vi "Kinect MVMT (state machine).vi"() -> ()   [LabVIEW 2011]
uses:
  Mouse Data Cluster.ctl
  <vilib>/vision/Image Controls.llb/IMAQ Image.ctl
  <vilib>/vision/NI_Vision_Development_Module.lvlib
panel:
  out "concatenated string 2":string
  out "Experiment Metadata":string
  in  "Experiment Metadata":i32(listbox)
  in  "Experiment File":path=path "C:/Users/Behavior Room/Desktop/Small Test.json"
  in  "Butt Position (pixels from left of image)":i32=10
  in  "Butt Threshold":dbl=150.0
  out "Mouse Tracked":bool
  in  "Flip?":bool
  out "Movement \nDecision":string
  out "Spine Contour":i32[](graph)
  in  "Milliseconds to wait between frames":u32
  in  "Gaussian Blur Kernel Size (From File)":i32=11
  in  "Distance to Camera Visible 3":cluster{dbl, dbl}(slide)={-1048.5759999999993, 2883.5840000000007} scale=-32768.0..32768.0
  in  "Divisor For Filter (From File)":sgl=0.5 min=0 max=1 step=0.1
  in  "Median Filter Size (From File)":i32=3 min=0 max=7
  in  "Path to Folder\nContaining TIFF Images":path=path "C:/Users/Behavior Room/Desktop/Recordings/Single Mouse"
  in  "History Length \nfor Head v Tail Determination":i32=100
  in  "Number of Erosion 2":i32=2
  in  "Selection Range 2":cluster{"Lower value":sgl, "Upper value":sgl}={"Lower value"=100.0, "Upper value"=32768.0}
  in  "Selection Parameters 2":T2(array[cluster])=[{"Measurement Parameter"=35, "Range Lower Value"=300, "Range Upper Value"=1500, "Range"=TRUE, "Measurement Type"=FALSE}] {"Measurement Parameter" items=["Center of Mass X", "Center of Mass Y", "First Pixel X", "First Pixel Y", "Bounding Rect Left", "Bounding Rect Top", "Bounding Rect Right", "Bounding Rect Bottom", "Max Feret Diameter Start X", "Max Feret Diameter Start Y", "Max Feret Diameter End X", "Max Feret Diameter End Y", "Max Horiz. Segment Length Left", "Max Horiz. Segment Length Right", "Max Horiz. Segment Length Row", "-", "Bounding Rect Width", "Bounding Rect Height", "Bounding Rect Diagonal", "Perimeter", "Convex Hull Perimeter", "Holes' Perimeter", "Max Feret Diameter", "Equivalent Ellipse Major Axis", "Equivalent Ellipse Minor Axis", "Equivalent Ellipse Minor Axis (Feret)", "Equivalent Rect Long Side", "Equivalent Rect Short Side", "Equivalent Rect Diagonal", "Equivalent Rect Short Side (Feret)", "Average Horiz. Segment Length", "Average Vert. Segment Length", "Hydraulic Radius", "Waddel Disk Diameter", "-", "Area", "Holes' Area", "Particle & Holes' Area", "Convex Hull Area", "Image Area", "-", "Number of Holes", "Number of Horiz. Segments", "Number of Vert. Segments", "-", "Orientation", "Max Feret Diameter Orientation", "-", "% Area/Image Area", "% Area/(Particle & Holes' Area)", "Ratio of Equivalent Ellipse Axes", "Ratio of Equivalent Rect Sides", "-", "Elongation Factor", "Compactness Factor", "Heywood Circularity Factor", "Type Factor", "-", "Sum X", "Sum Y", "Sum XX", "Sum XY", "Sum YY", "Sum XXX", "Sum XXY", "Sum XYY", "Sum YYY", "-", "Moment of Inertia XX", "Moment of Inertia XY", "Moment of Inertia YY", "Moment of Inertia XXX", "Moment of Inertia XXY", "Moment of Inertia XYY", "Moment of Inertia YYY", "Norm. Moment of Inertia XX", "Norm. Moment of Inertia XY", "Norm. Moment of Inertia YY", "Norm. Moment of Inertia XXX", "Norm. Moment of Inertia XXY", "Norm. Moment of Inertia XYY", "Norm. Moment of Inertia YYY", "Hu Moment 1", "Hu Moment 2", "Hu Moment 3", "Hu Moment 4", "Hu Moment 5", "Hu Moment 6", "Hu Moment 7"]}
  out "Extracted Diff Image":T3(plugin-control)
  in  "Median Filter Size 2":i32=3 min=0 max=7
  in  "Divisor 2":sgl=0.5 min=0 max=1 step=0.1
  in  "Distance to Camera Visible 2":cluster{dbl, dbl}(slide)={-1048.5759999999993, 2883.5840000000007} scale=-32768.0..32768.0
  out "Extracted Image":T3(plugin-control)
  in  "Height":i32=80
  in  "Width":i32=80
  in  "Acquire Background":bool
  in  "Number of Frames To Average\nfor Background Image":i32=200 min=1 max=1000
  out "Heat Map":T3(plugin-control)
  out "Mask":T3(plugin-control)
  in  "Gaussian Blur Kernel Size":i32=11
  in  "Distance to Camera Visible":cluster{dbl, dbl}(slide)={-4718.592, 13369.344000000001} scale=-32768.0..32768.0
  in  "Post Extraction Limit":cluster{dbl, dbl}(slide)={48.0, 888.0} scale=-3000.0..3000.0
  in  "Divisor":sgl=0.5 min=0 max=1 step=0.1
  in  "Median Filter Size":i32=5 min=0 max=7
  out "Diff Image":T3(plugin-control)
  out "Raw Image":T3(plugin-control)
  in  "OK":bool
  # "Misc"
  # "Preprocessing"
  # "Particle Finding"
  # "Head vs. Tail Determination"
  # "Difference Image Processing"
  # "File Saving"
  # "Playback"
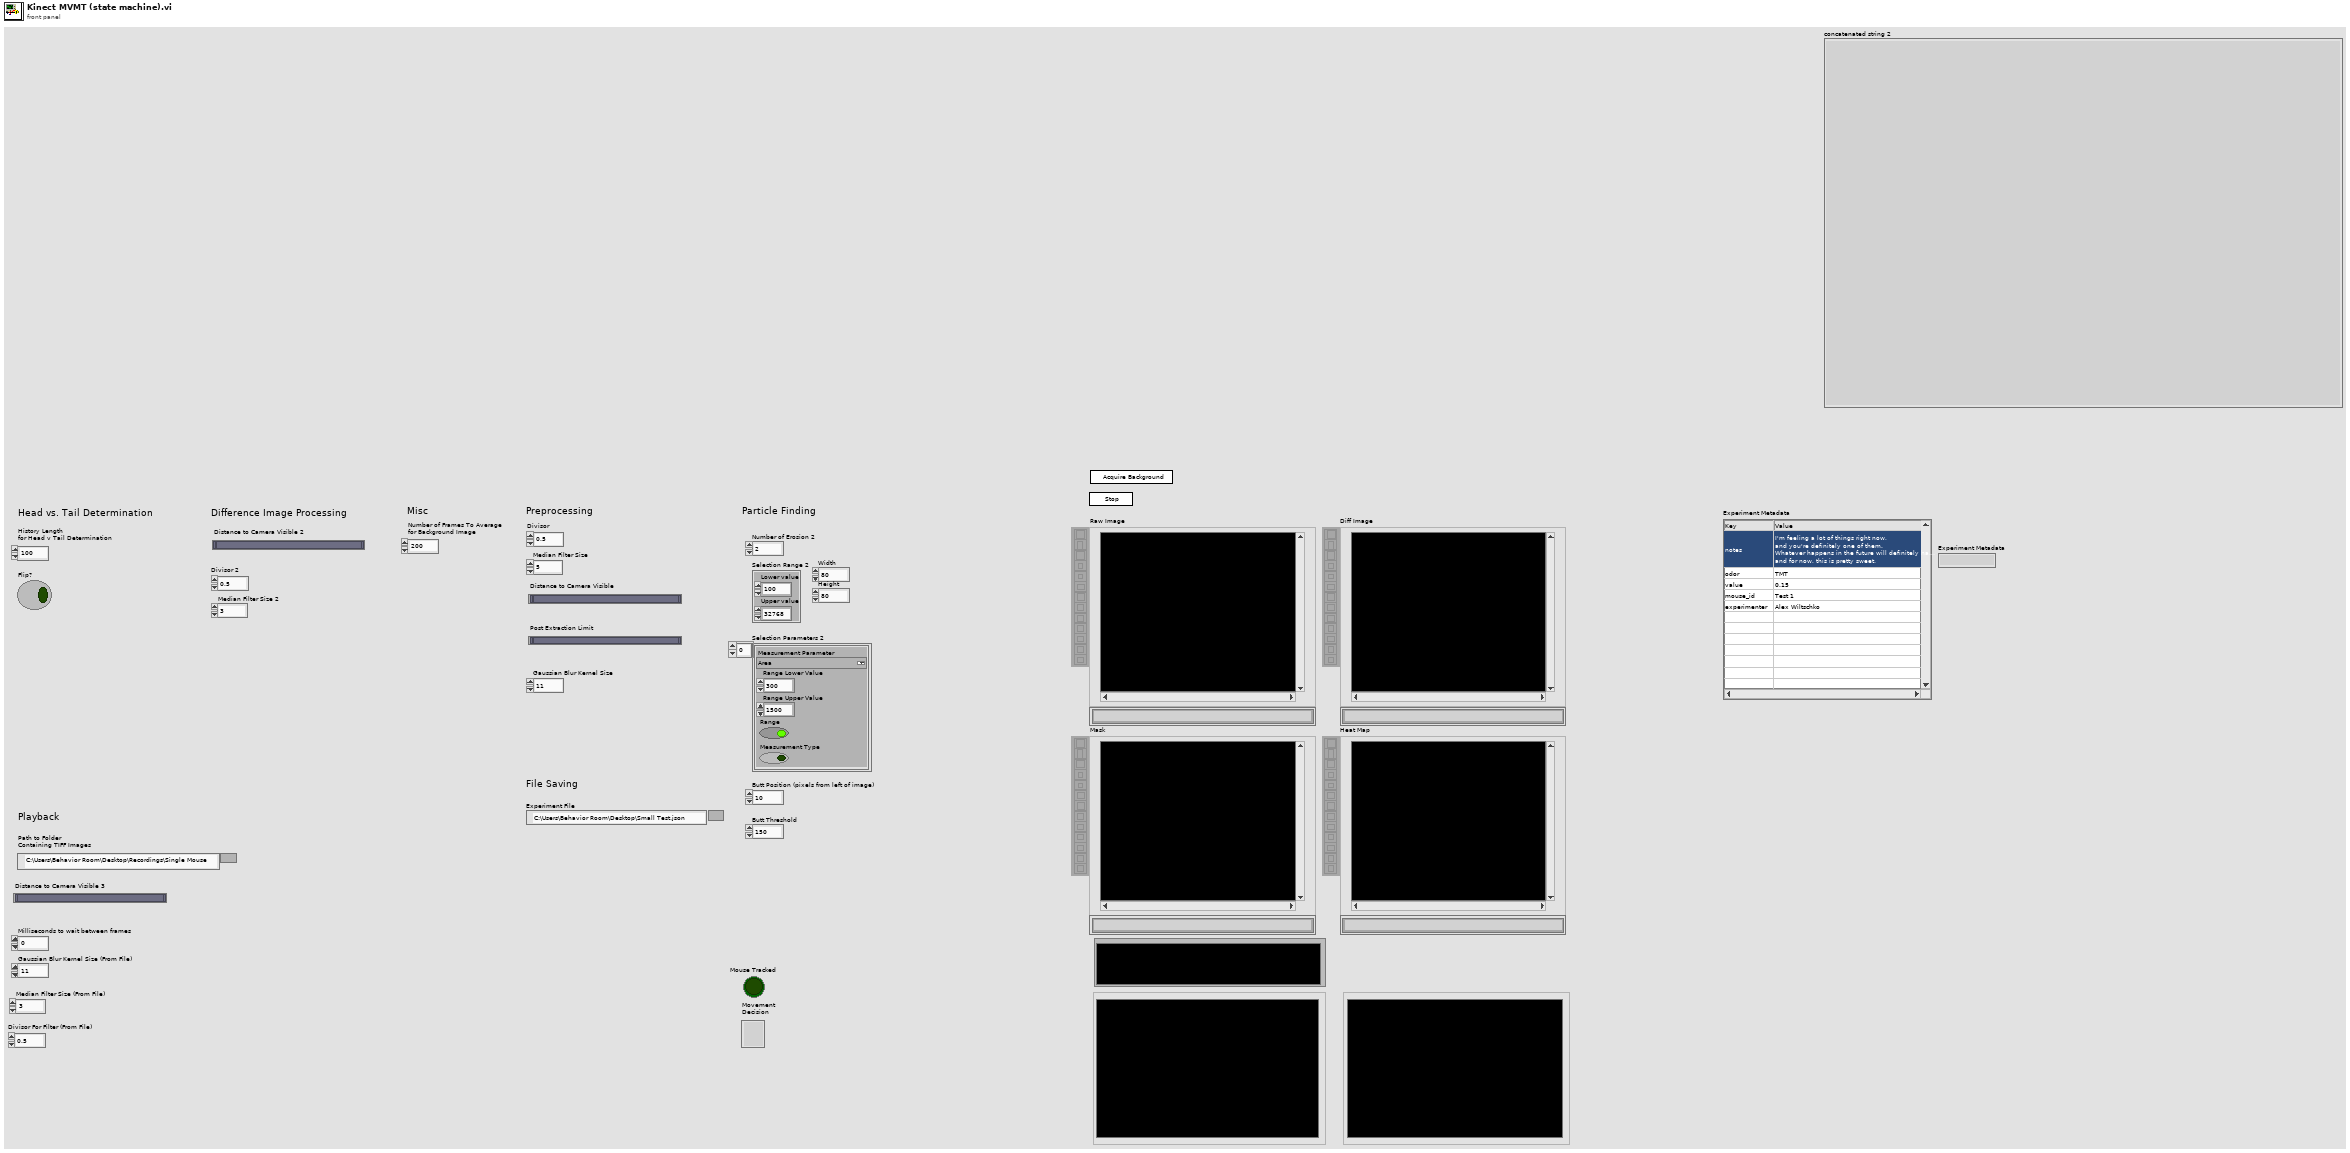
[diagram p1: front panel]
types:
  T1 = typedef "Particle Parameters" = i32
  T2 = cluster{"Measurement Parameter":T1, "Range Lower Value":i32, "Range Upper Value":i32, "Range":bool, "Measurement Type":bool}[]
  T3 = typedef "IMAQ Image.ctl" = refnum<image>
  T4 = enum32{"invalid app kind", "Development System", "Run Time System", "Student Edition", "Embedded LabVIEW", "Evaluation", "Custom"}
  T5 = typedef "Mouse Data Cluster.ctl" = cluster{"Mouse Image":T3, "Mouse Difference Image":T3, "Angle":i32, "Spine Contour":i32[], "Outline Contour":i32[][], "Timestamp":dbl, "Height":i32, "Width":i32, "Length":i32, "Area":sgl, "POI Offsets":cluster{"X":i32, "Y":i32, "Distance":i32, "POI Name":string}[], "Frame ID":i16, "Centroid X":i32, "Centroid Y":i32, "Head X":i32, "Head Y":i32, "Tail X":i32, "Tail Y":i32}
  T6 = enum32{"Invalid", "Standard", "Closed", "Hidden", "Minimized", "Maximized"}
  T7 = enum32{"Average", "Min", "Max", "Clear  if < ", "Clear  if < or =", "Clear  if =", "Clear  if > or =", "Clear  if >"}
  T8 = enum16{"open", "replace", "create", "open or create", "replace or create", "replace or create with confirmation"}
  T9 = cluster{"Core":cluster{"Current VI Reference":refnum<vi>, "Close Panel on Exit?":bool}, "Background Image":T3, "Background Image Path":path, "Processed Background Image":T3, "Kinect Acquisition Queue":refnum<queue>, "Raw Image":T3, "Difference Image":T3, "Processed Image":T3, "Processed Diff Image":T3, "Particle Mask":T3, "Occupancy Map":T3, "Timestamp":i32, "Mouse Data":T5, "Particle Report":cluster{"Area":dbl, "Number of Holes":dbl, "Bounding Rect":cluster{"Left":dbl, "Top":dbl, "Right":dbl, "Bottom":dbl}, "Center of Mass":cluster{"X":dbl, "Y":dbl}, "Orientation":dbl, "Dimensions":cluster{"Width":dbl, "Height":dbl}}, "Mouse Identified":bool, "refnum out":refnum<file>}
  T10 = cluster{"Area":dbl, "Number of Holes":dbl, "Bounding Rect":cluster{"Left":dbl, "Top":dbl, "Right":dbl, "Bottom":dbl}, "Center of Mass":cluster{"X":dbl, "Y":dbl}, "Orientation":dbl, "Dimensions":cluster{"Width":dbl, "Height":dbl}}
  T11 = cluster{"Mouse Image":T3, "Mouse Difference Image":T3, "Position":cluster{"X":i32, "Y":i32}, "Angle":i32, "Spine Contour":i32[], "Outline Contour":i32[][], "Timestamp":i32, "Height":i32, "Width":i32, "Length":i32, "Area":i32, "Perimeter":i32, "POI Offsets":cluster{"X":i32, "Y":i32, "Distance":i32, "POI Name":string}[]}
  T12 = cluster{"Current VI Reference":refnum<vi>, "Close Panel on Exit?":bool}
  T13 = typedef "Image Type" = u32
  T14 = cluster{"Area":dbl, "Number of Holes":dbl, "Bounding Rect":cluster{"Left":dbl, "Top":dbl, "Right":dbl, "Bottom":dbl}, "Center of Mass":cluster{"X":dbl, "Y":dbl}, "Orientation":dbl, "Dimensions":cluster{"Width":dbl, "Height":dbl}}[]
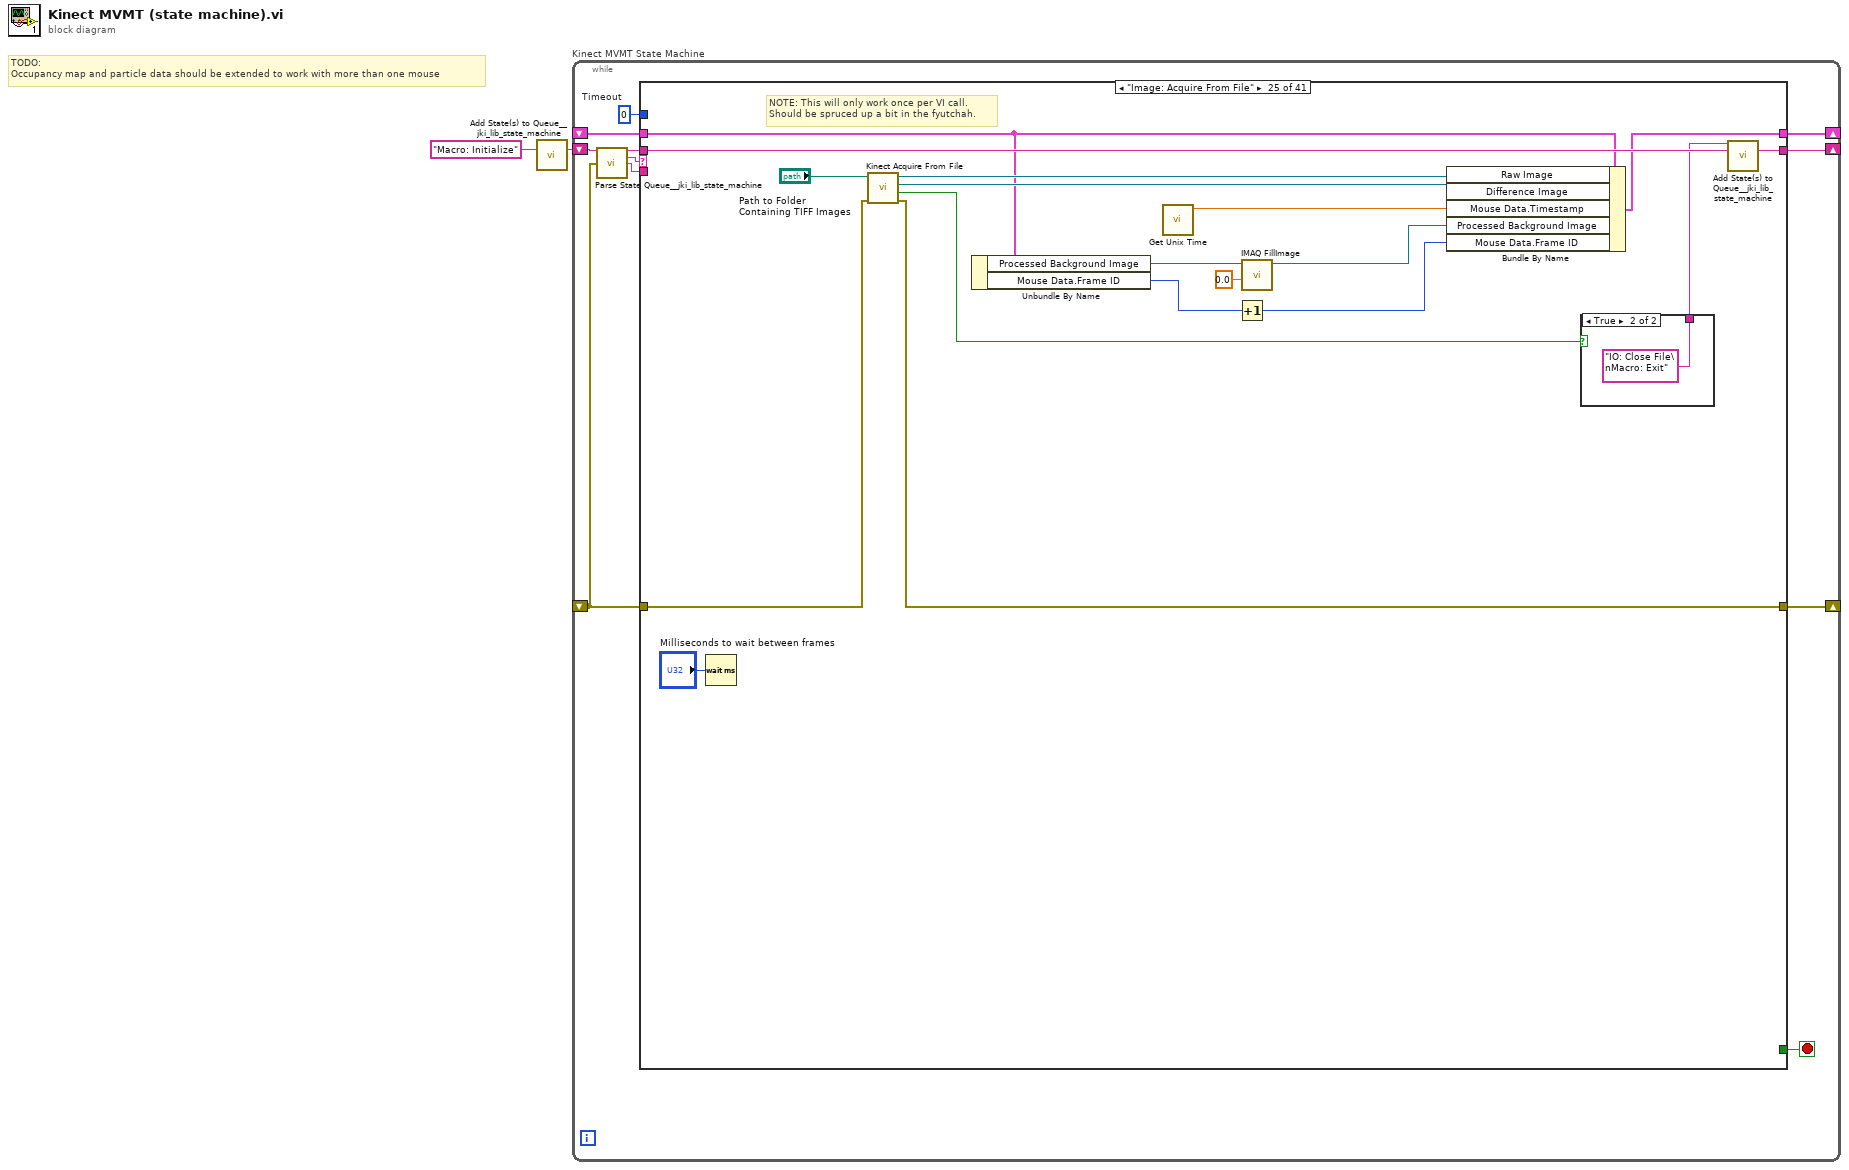
[diagram p0: block diagram]
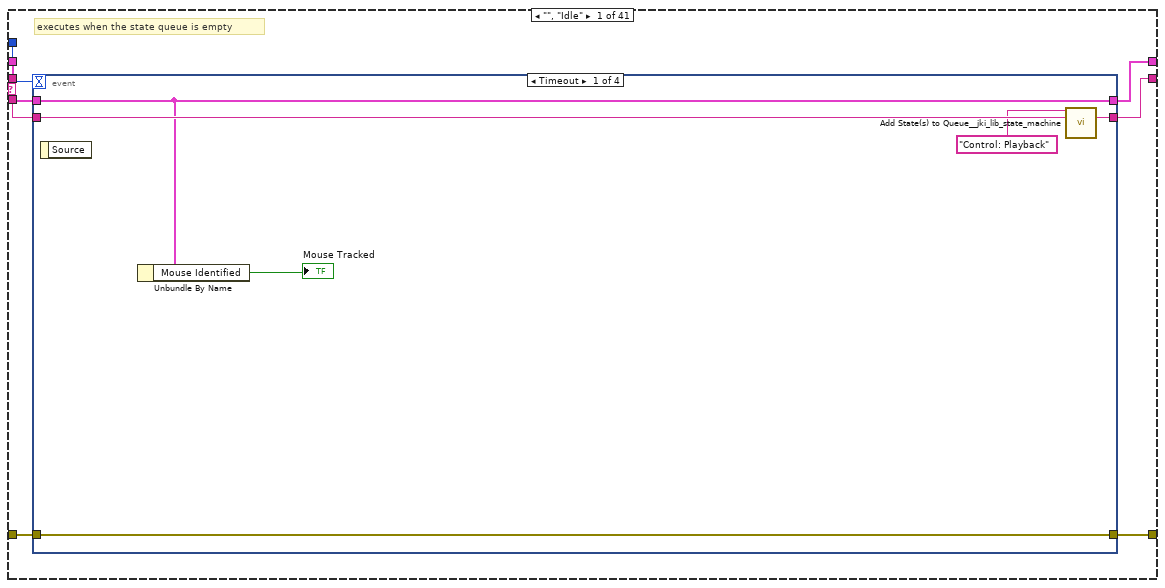
[diagram p2: hidden frame]
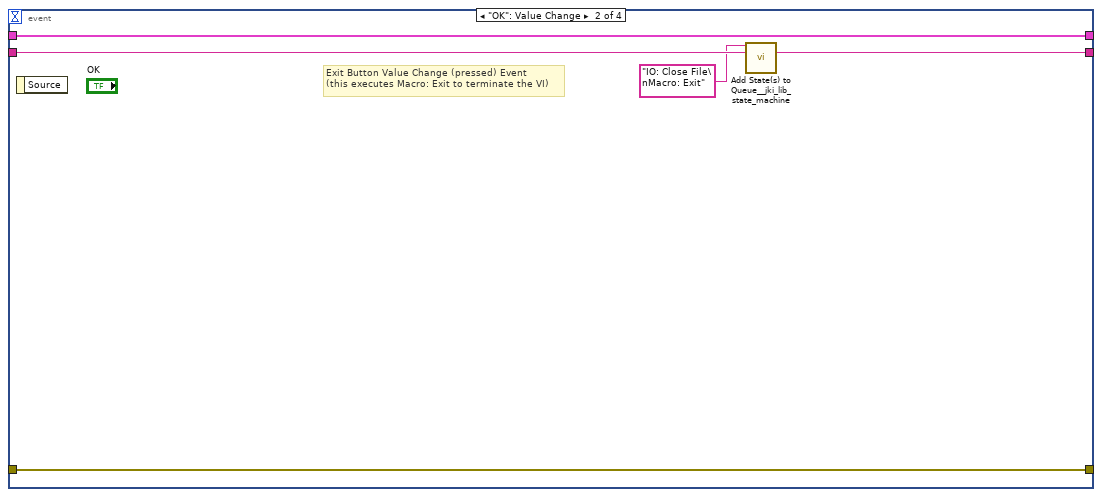
[diagram p3: hidden frame]
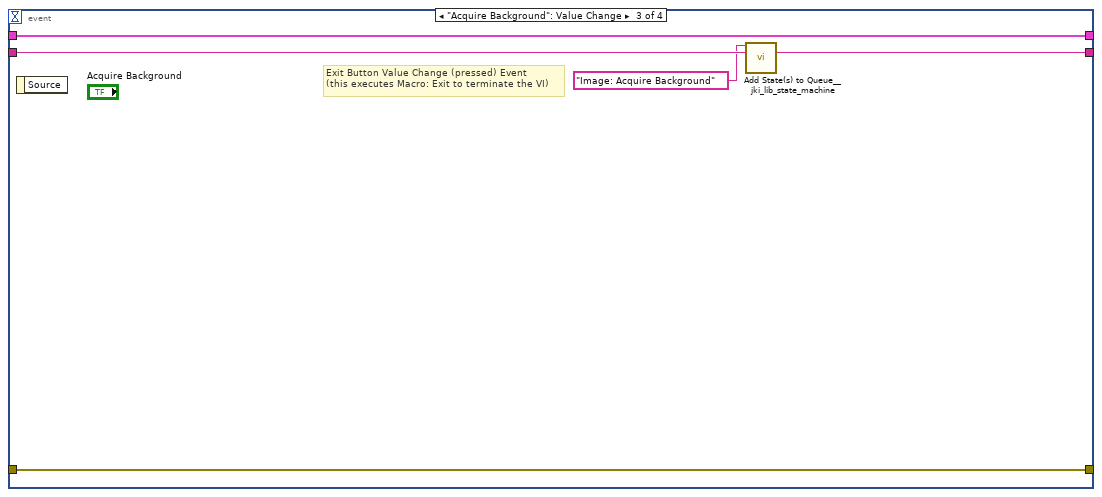
[diagram p4: hidden frame]
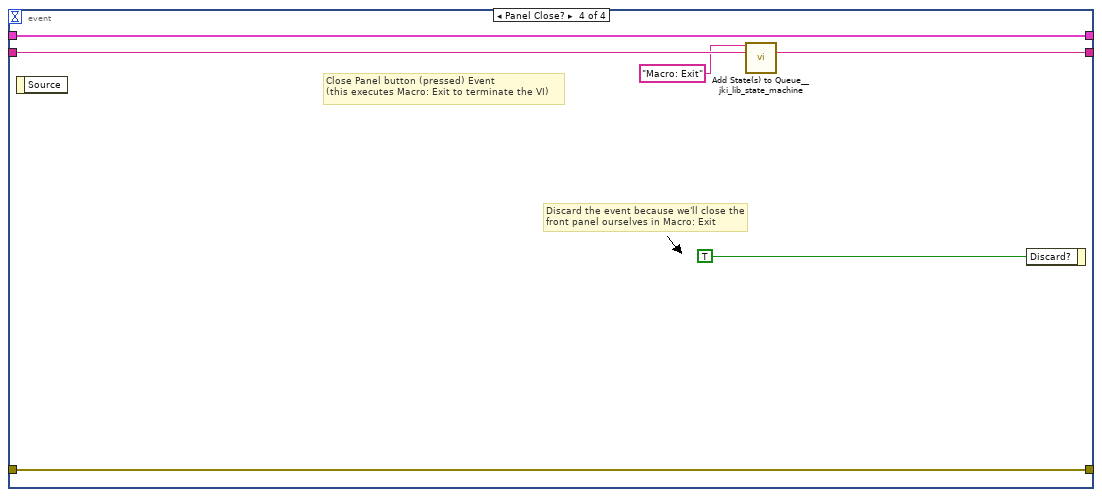
[diagram p5: hidden frame]
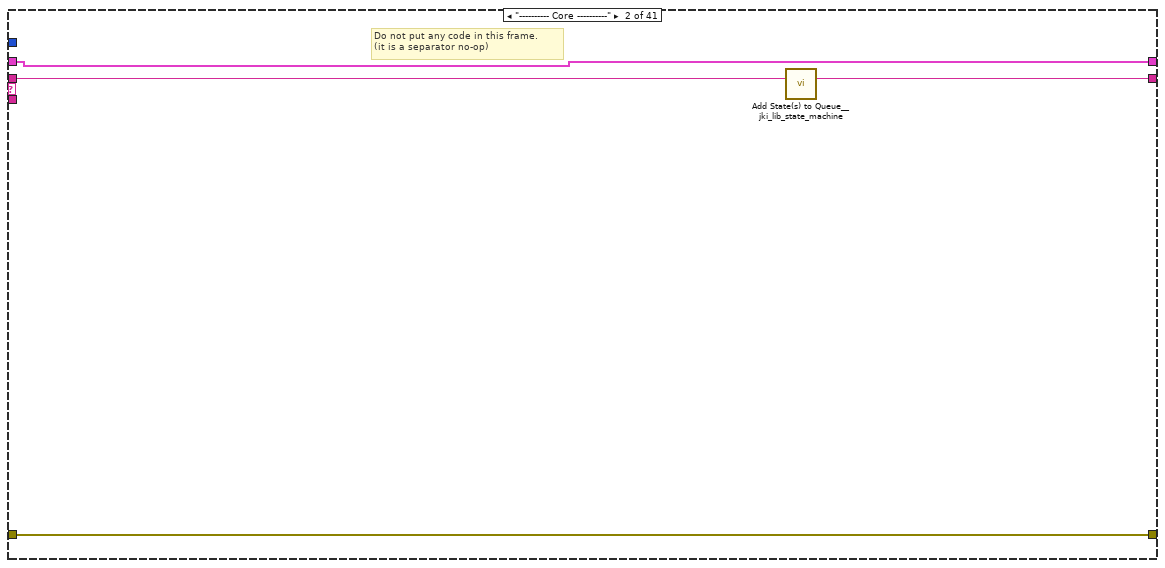
[diagram p6: hidden frame]
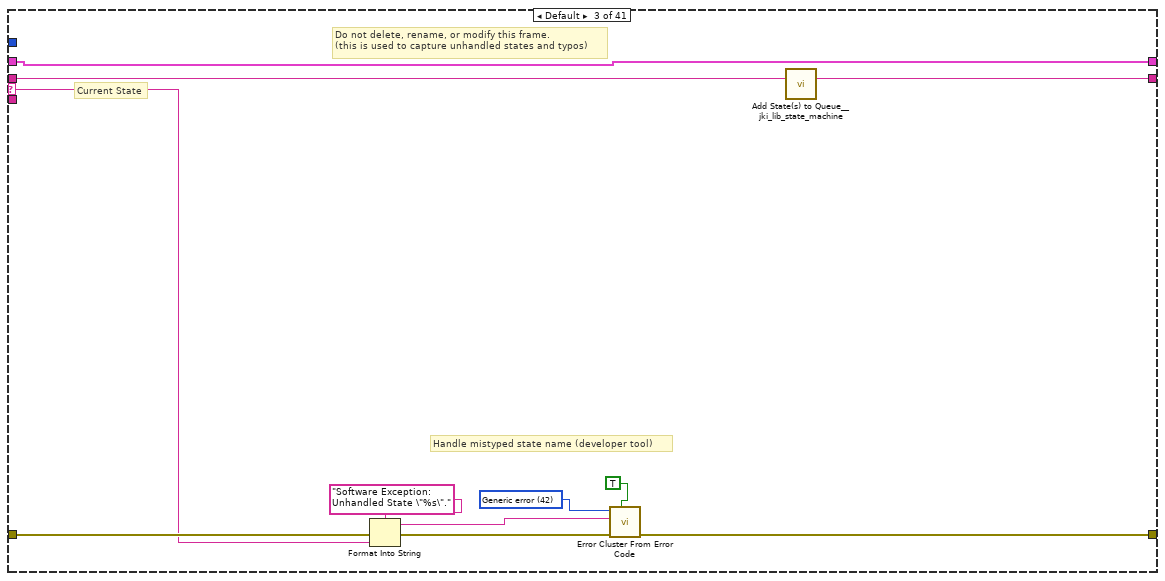
[diagram p7: hidden frame]
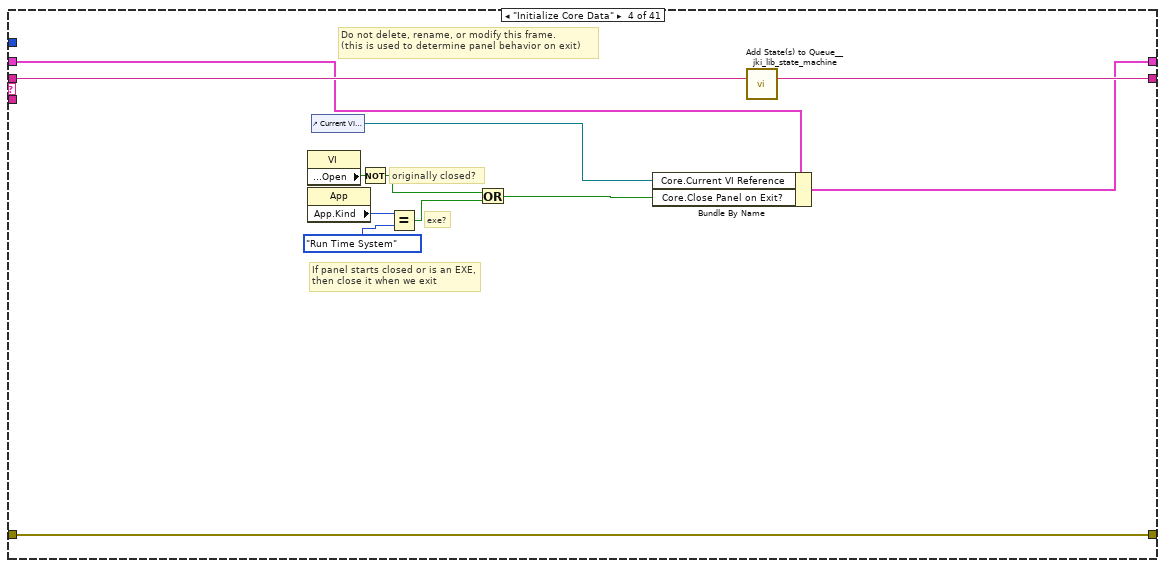
[diagram p8: hidden frame]
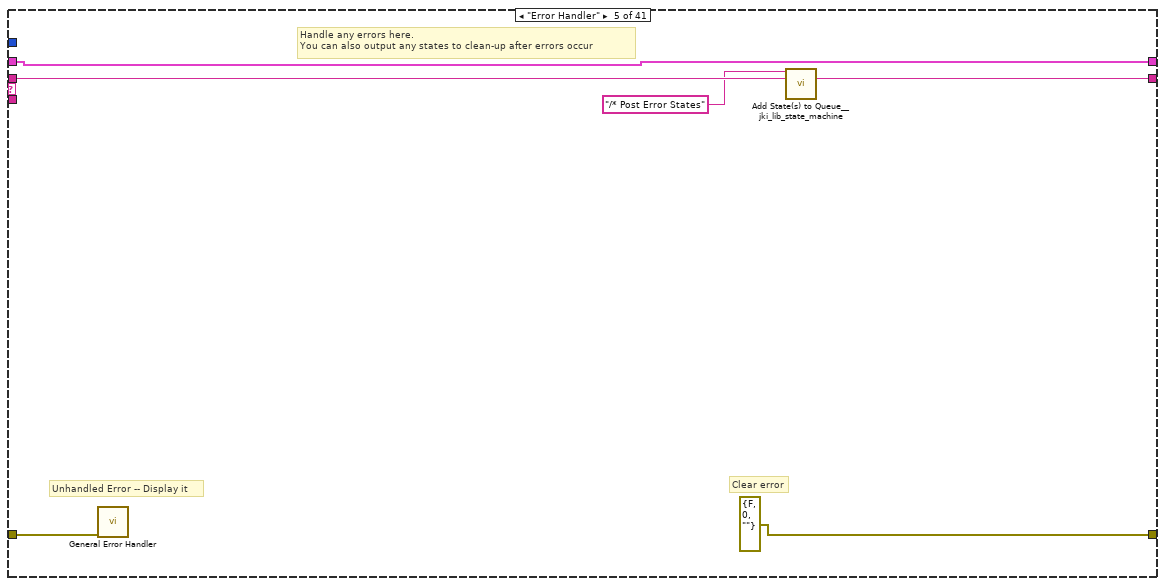
[diagram p9: hidden frame]
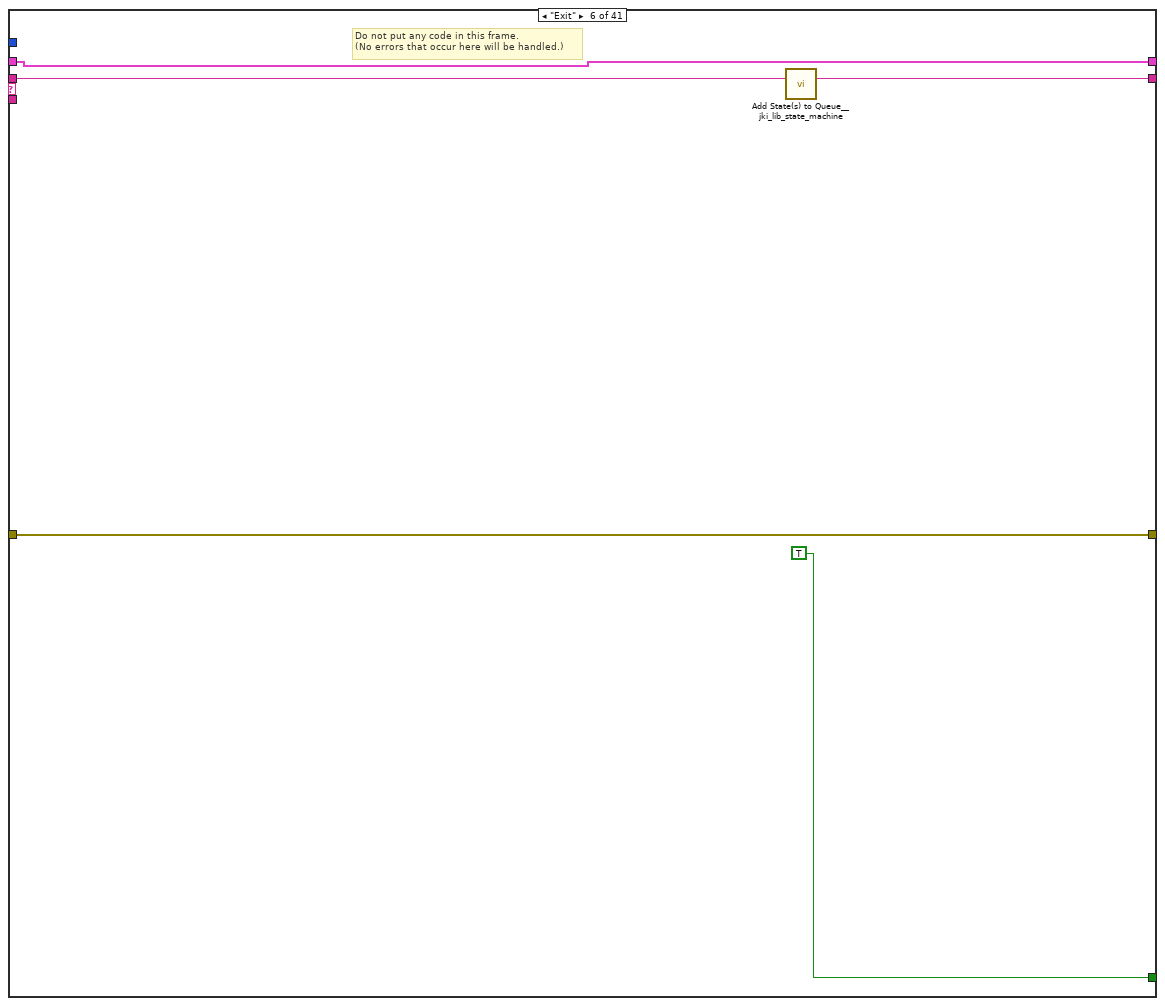
[diagram p10: hidden frame]
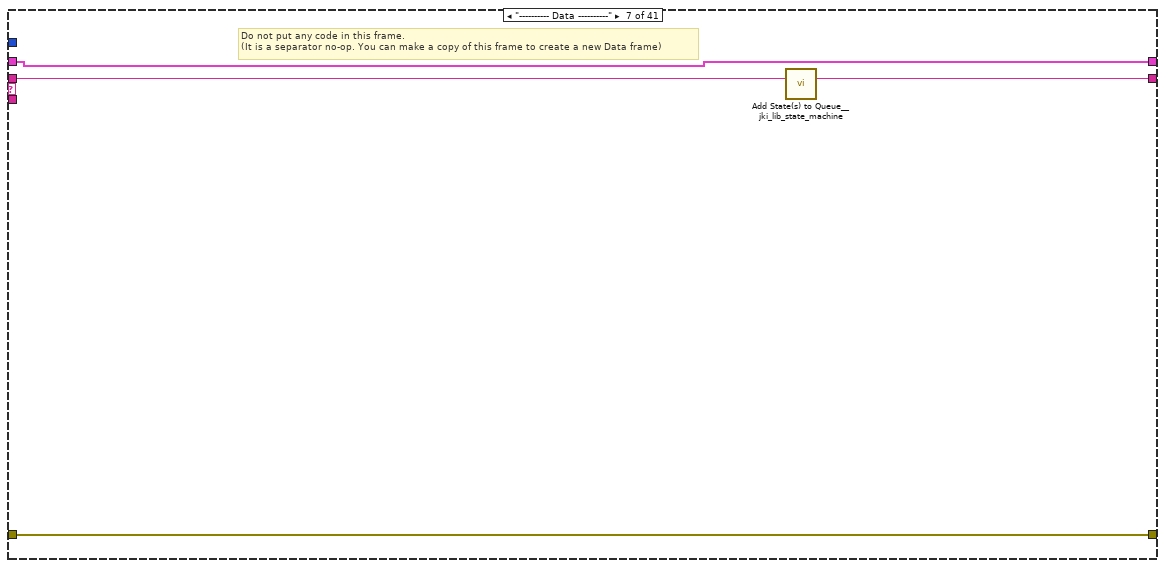
[diagram p11: hidden frame]
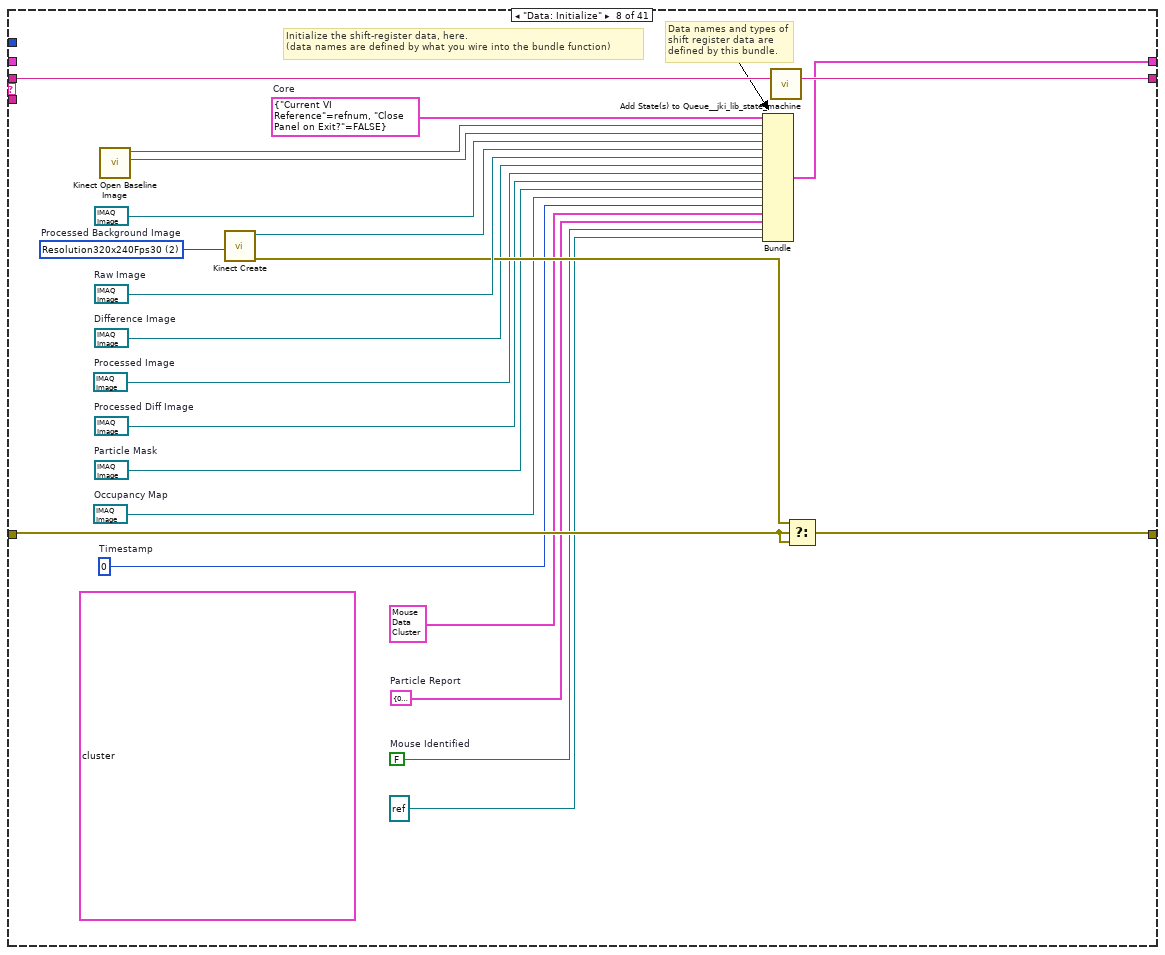
[diagram p12: hidden frame]
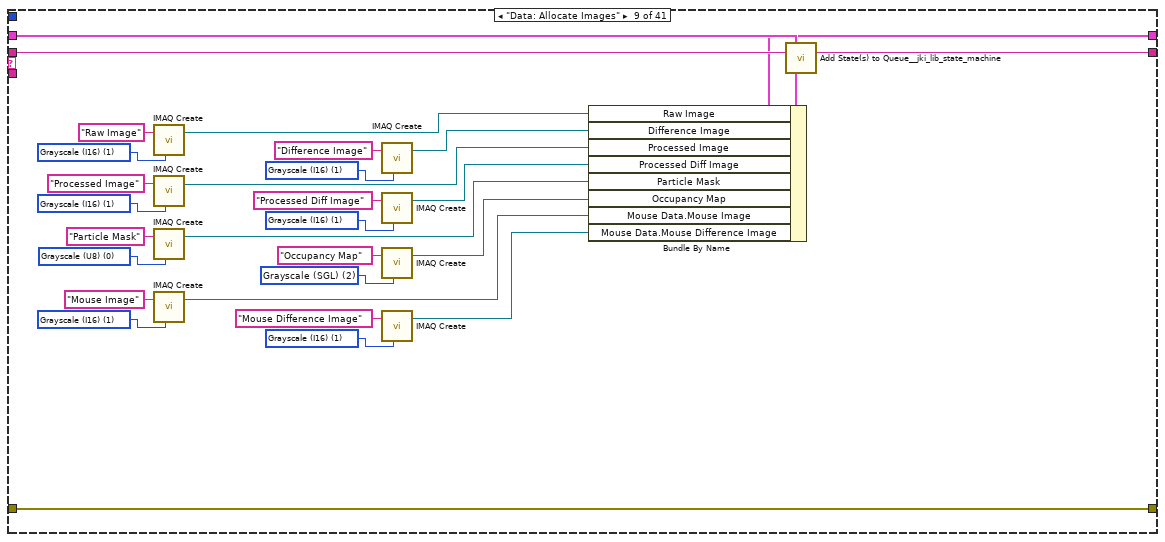
[diagram p13: hidden frame]
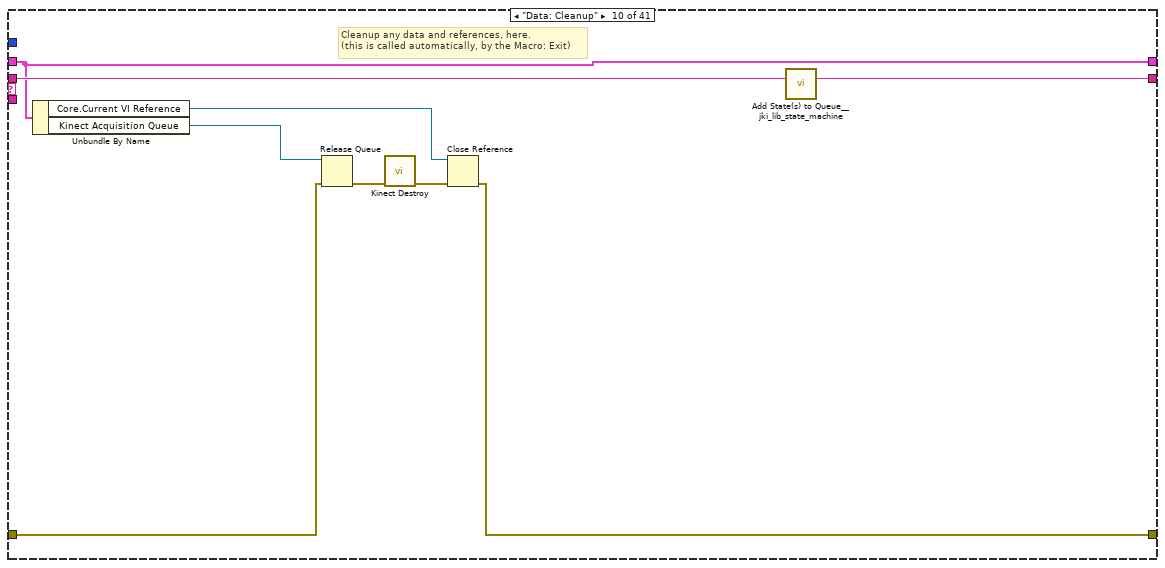
[diagram p14: hidden frame]
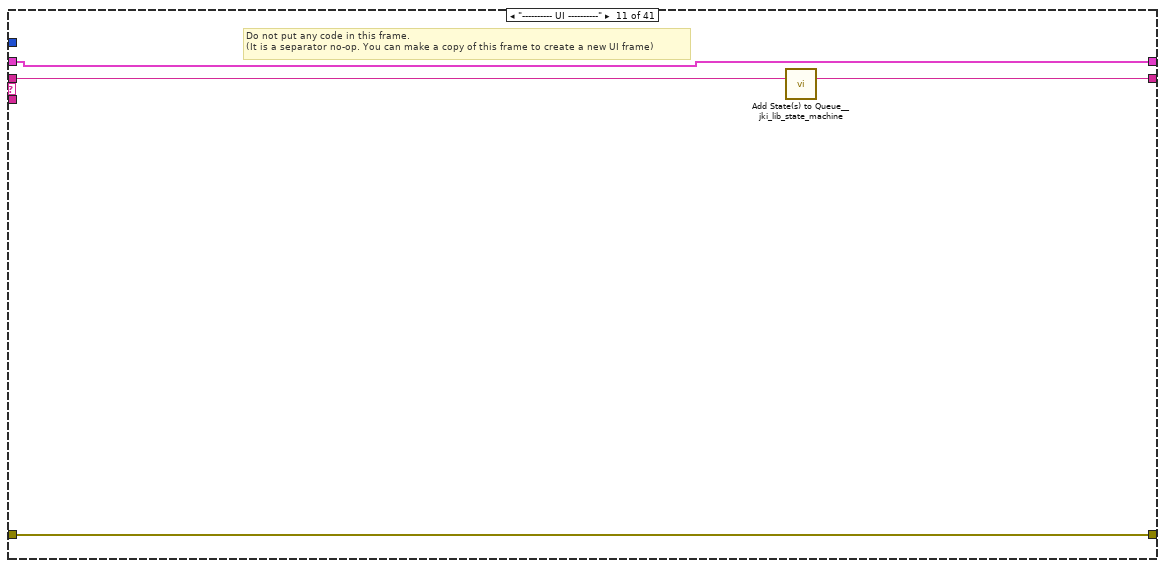
[diagram p15: hidden frame]
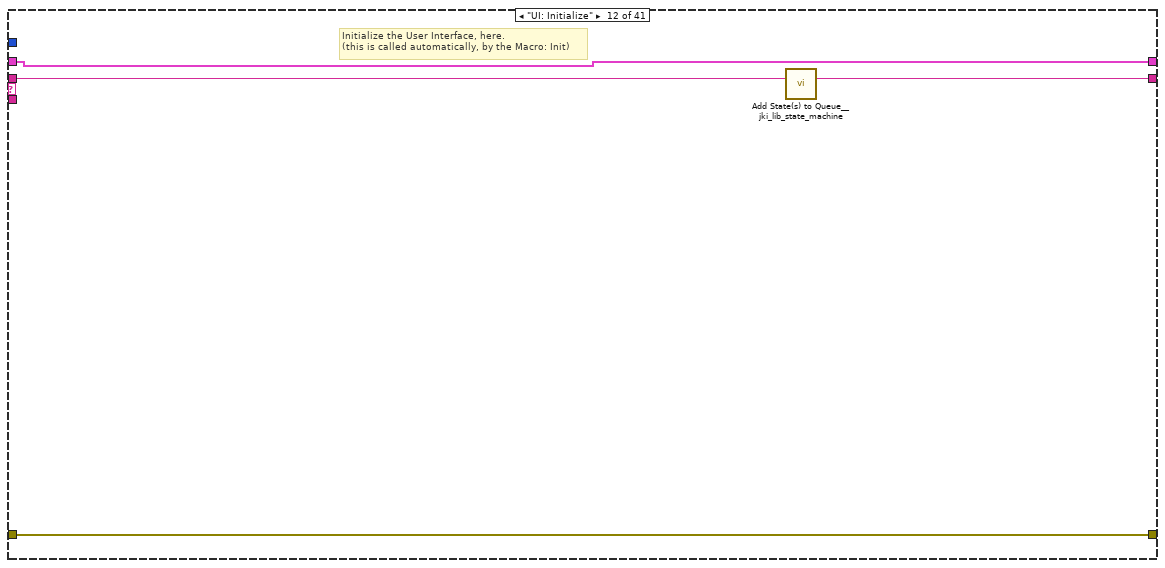
[diagram p16: hidden frame]
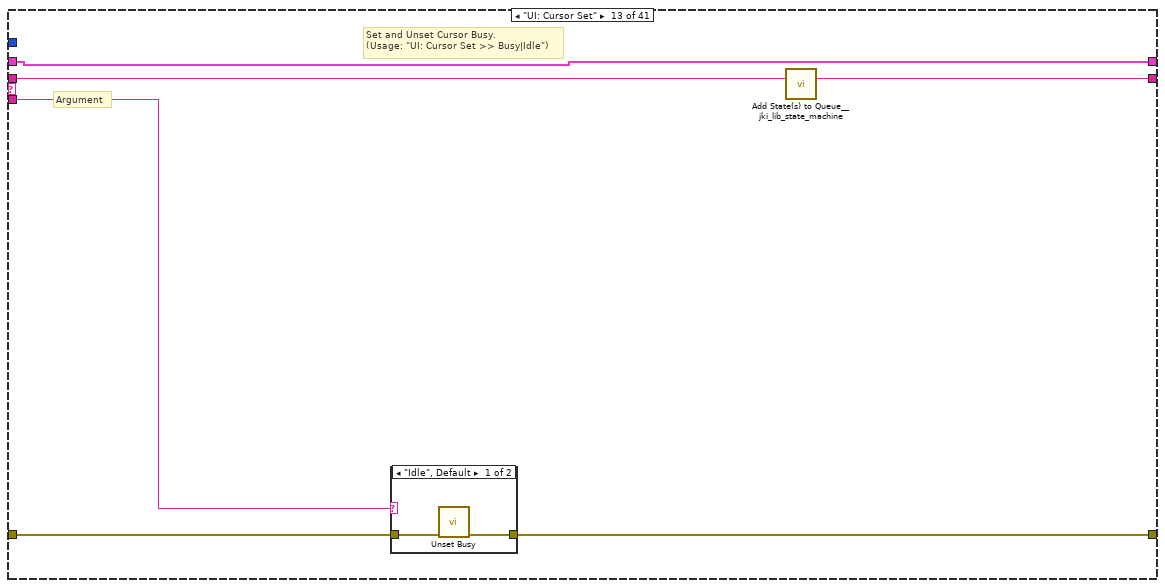
[diagram p17: hidden frame]
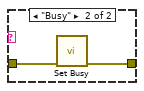
[diagram p18: hidden frame]
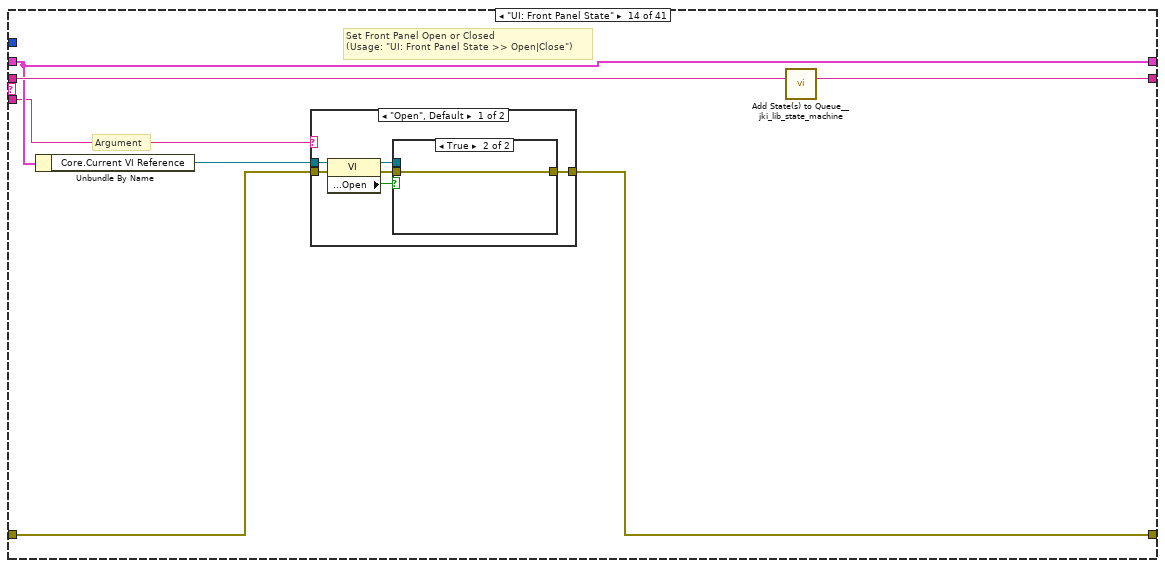
[diagram p19: hidden frame]
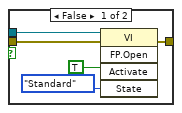
[diagram p20: hidden frame]
diagram:
  # "TODO:\nOccupancy map and particle data should be extended to work with more than one mouse"
  n1 = call <vilib>:"Add State(s) to Queue__jki_lib_state_machine.vi"("State(s) in (\"\")"="Macro: Initialize") -> ("States Out"=w2:string)  [unwired: 14 in]
  n2 = while "Kinect MVMT State Machine" {
    shift-right: [w6] -> _
    shift-left: _ -> [w5]
    shift-right: [w9] -> _
    shift-left: _ -> [w3]
    shift-right: [w8] -> _
    shift-left: w2 -> [w10]
    stop <- w7 stop-if-true
    w4 = 0  # Timeout
    n3 = call <vilib>:"Parse State Queue__jki_lib_state_machine.vi"("State Queue"=w10, "Error In (no error)"=w3) -> ("Remaining States"=w12:string, "Current State"=w13:string, "Arguments"=w11:string)  [unwired: 11 in]
    n4 = case shown="\"Image: Acquire From File\"" w13 {
      selector: w13 -> [_ _ w47 _ _ _ _ _ _ _ _ _ _ _ _ _ _ _ _ _ _ _ _ _ _ _ _ _ _ _ _ _ _ _ _ _ _ _ _ _ _]
      tunnel: w12 -> [w20 w46 w51 w69 w75 w80 w84 w107 w136 w145 w149 w153 w159 w170 w196 w201 w211 w215 w220 w225 w230 _ w240 w252 w270 w295 w311 w329 w348 w387 w400 w430 w454 w464 w508 w522 w535 w547 w557 w571 w589]
      tunnel: w11 -> [_ _ _ _ _ _ _ _ _ _ _ _ w154 w164 _ _ _ _ _ _ _ _ _ _ _ _ _ _ _ _ _ _ _ _ _ _ _ _ _ _ _]
      tunnel: w5 -> [w18 w43 w49 w60 w72 w78 w81 _ w133 w141 w146 w151 w157 w166 w193 w198 w208 w212 w217 w222 w227 w234 w237 w249 w260 w283 w304 w320 w337 w371 w389 w426 w452 w462 w499 w515 w533 w544 w553 w568 w586]
      tunnel: [w17 w44 w53 w66 errorcluster {"status"=FALSE, "code"=0, "source"=""} ("error out") w77 w82 w98 w134 w142 w147 w150 w155 w167 w194 w199 w209 w213 w218 w223 w228 w235 w238 w243 w263 w280 w303 w322 w346 w382 w398 w428 w448 w457 w506 w520 w523 w545 w555 w569 w587] -> w9
      tunnel: w3 -> [w16 w44 w52 w66 w71 w77 w82 w96 w134 w138 w147 w150 w156 w168 w194 w199 w209 w213 w218 w223 w228 w235 w238 w244 w264 w279 w297 w323 w346 w384 w398 w428 w449 w456 w506 w520 w529 w545 w555 w569 w587]
      tunnel: [w19 w45 w50 w68 w74 w79 w83 w106 w135 w144 w148 w152 w158 w169 w195 w200 w210 w214 w219 w224 w229 w236 w239 w251 w269 w294 w310 w328 w347 w386 w399 w429 w453 w463 w507 w521 w534 w546 w556 w570 w588] -> w8
      tunnel: [_ _ _ _ _ TRUE _ _ _ _ _ _ _ _ _ _ _ _ _ _ _ _ _ _ _ _ _ _ _ _ _ _ _ _ _ _ _ _ _ _ _] -> w7
      tunnel: [w15 w43 w49 w67 w72 w78 w81 w105 w132 w141 w146 w151 w157 w166 w193 w198 w208 w212 w217 w222 w227 w233 w237 w248 w268 w293 w309 w318 w336 w385 w388 w425 w451 w461 w499 w514 w532 w544 w552 w568 w586] -> w6
      tunnel: w4 -> [w14 _ _ _ _ _ _ _ _ _ _ _ _ _ _ _ _ _ _ _ _ _ _ _ _ _ _ _ _ _ _ _ _ _ _ _ _ _ _ _ _]
      frame "", "Idle" {
        # "executes when the state queue is empty"
        n5 = event shown="[0] Timeout" {
          selector: _ -> [_ _ _ _]
          dyn-events: _ -> [_ _ _ _]
          timeout: w14 -> [_ _ _ _]
          tunnel: w20 -> [w24 w31 w36 w42]
          tunnel: [w26 w30 w35 w41] -> w19
          tunnel: w18 -> [w21 w27 w33 w39]
          tunnel: [w25 w29 w34 w40] -> w17
          tunnel: w16 -> [w25 w29 w34 w40]
          tunnel: [w21 w27 w33 w39] -> w15
          event Timeout {
            n6 = event-data() -> ()  [unwired: 1 in, 1 out]
            n7 = Unbundle By Name(w21) -> ("Mouse Identified"=→"Mouse Tracked":bool)
            n8 = call <vilib>:"Add State(s) to Queue__jki_lib_state_machine.vi"("State(s) in Front (\"\")"="Control: Playback" ("State(s) in Front (\"\")"), "State(s) in (\"\")"=w24) -> ("States Out"=w26:string)  [unwired: 13 in]
          }
          event "OK": Value Change {
            # "Exit Button Value Change (pressed) Event\n(this executes Macro: Exit to terminate the VI)"
            n9 = event-data() -> ()  [unwired: 1 in, 1 out]
            n10 = call <vilib>:"Add State(s) to Queue__jki_lib_state_machine.vi"("State(s) in Front (\"\")"="IO: Close File\nMacro: Exit", "State(s) in (\"\")"=w31) -> ("States Out"=w30:string)  [unwired: 13 in]
          }
          event "Acquire Background": Value Change {
            # "Exit Button Value Change (pressed) Event\n(this executes Macro: Exit to terminate the VI)"
            n11 = event-data() -> ()  [unwired: 1 in, 1 out]
            n12 = call <vilib>:"Add State(s) to Queue__jki_lib_state_machine.vi"("State(s) in Front (\"\")"="Image: Acquire Background" ("State(s) in Front (\"\")"), "State(s) in (\"\")"=w36) -> ("States Out"=w35:string)  [unwired: 13 in]
          }
          event Panel Close? {
            # "Discard the event because we'll close the front panel ourselves in Macro: Exit"
            # "Close Panel button (pressed) Event\n(this executes Macro: Exit to terminate the VI)"
            n13 = event-data() -> ()  [unwired: 1 in, 1 out]
            n14 = call <vilib>:"Add State(s) to Queue__jki_lib_state_machine.vi"("State(s) in Front (\"\")"="Macro: Exit", "State(s) in (\"\")"=w42) -> ("States Out"=w41:string)  [unwired: 13 in]
            n15 = event-data("Discard?"=TRUE) -> ()  [unwired: 1 in, 1 out]
          }
        }
      }
      frame "---------- Core ----------" {
        # "Do not put any code in this frame.\n(it is a separator no-op)"
        n16 = call <vilib>:"Add State(s) to Queue__jki_lib_state_machine.vi"("State(s) in (\"\")"=w46) -> ("States Out"=w45:string)  [unwired: 14 in]
      }
      frame Default {
        w56 = 42 items=["No error", "Argument error", "Memory is full", "Out of zone", "End of file", "File already open", "Generic file I/O error", "File not found", "File permission error", "Disk is full", "Duplicate path", "Too many files open", "System feature not enabled", "Resource file not found", "Cannot add resource", "Resource not found", "Image not found", "Image memory error", "Pen does not exist", "Config type invalid", "Config token not found", "Config parse error", "Config memory error", "Bad external code format", "Bad external code offset", "External code not present", "Null window", "Destroy window error", "Null menu", "Print aborted", "Bad print record", "Print driver error", "Windows error during printing", "Memory error during printing", "Print dialog error", "Generic print error", "Invalid device refnum", "Device not found", "Device parameter error", "Device unit error", "Cannot open device", "Device call aborted", "Generic error", "Cancelled by user", "Object ID too low", "Object ID too high", "Object not in heap", "Unknown heap", "Unknown object (invalid DefProc)", "Unknown object (DefProc not in table)", "Message out of range", "Invalid (null) method", "Unknown message", "Manager call not supported", "Bad address", "Network operation in progress", "Network operation timed out", "Connection is busy", "Network attribute not supported", "Network error", "Address in use", "System out of memory", "Connection aborted", "Connection refused", "Not connected", "Already connected", "Connection closed", "Initialization error (interapplication manager)", "Bad occurrence", "Wait on unbound occurrence handler", "Occurrence queue overflow", "Datalog type conflict", "Unused", "Unrecognized type (interapplication manager)", "Memory corrupt", "Failed to make temporary DLL", "Old CIN version", "Drag socket not found", "Failed to load drop-object", "Failed to register OLE object", "Failed to release OLE object", "Format specifier type mismatch", "Unknown format specifier", "Too few format specifiers", "Too many format specifiers", "Scan failed", "Newer CIN version", "Error converting to variant", "Runtime menu error", "Password tampered", "Variant attribute not found", "Incompatible variant data type", "Event data is not available", "Event Store is not present", "Occurrence is not found", "Event Queue is not created", "Event info is not available", "Refnum passed is NULL", "Error retrieving Class GUID", "Error retrieving CoClass GUID", "Error retrieving TypeLib GUID.", "Bad built application magic bytes.", "Specific driver is different from the specific driver associated with the Logical Name.", "There is no session opened to the class driver.", "Max Error", "MAX - Error with config objects", "MAX - Error loading configuration", "MAX - Group not supported"]
        # "Current State"
        # "Do not delete, rename, or modify this frame.\n(this is used to capture unhandled states and typos)"
        # "Handle mistyped state name (developer tool)"
        n17 = Format Into String(format string="Software Exception: Unhandled State \"%s\"." ("message"), error in=w52, w47) -> (resulting string=w55:string, error out=w54:errorcluster)  [unwired: 1 in]
        n18 = call <vilib>:"Error Cluster From Error Code.vi"("show call chain? (False)"=TRUE, "error in (no error)"=w54, "error message (\"\")"=w55, "error code (0)"=w56) -> ("error out"=w53:errorcluster)  [unwired: 5 in]
        n19 = call <vilib>:"Add State(s) to Queue__jki_lib_state_machine.vi"("State(s) in (\"\")"=w51) -> ("States Out"=w50:string)  [unwired: 14 in]
      }
      frame "Initialize Core Data" {
        # "Do not delete, rename, or modify this frame.\n(this is used to determine panel behavior on exit)"
        # "originally closed?"
        # "exe?"
        # "If panel starts closed or is an EXE, then close it when we exit"
        n20 = property class="VI"() -> ("Front Panel.Open"=w65:bool)  [unwired: 2 in, 2 out]
        n21 = property class="App"() -> ("App.Kind"=w64:T4)  [unwired: 2 in, 2 out]
        n22 = control-ref of="Current VI Reference"() -> (w58:refnum<vi>)
        n23 = Not(x=w65) -> (.not. x?=w62:bool)
        n24 = Equal?(x=w64, y=T4."Run Time System" ("Application:Kind")) -> (x = y?=w61:bool)
        n25 = Or(x=w62, y=w61) -> (x .or. y?=w59:bool)
        n26 = Bundle By Name(cluster=w60, "Core.Current VI Reference"=w58, "Core.Close Panel on Exit?"=w59) -> (w67:T9)
        n27 = call <vilib>:"Add State(s) to Queue__jki_lib_state_machine.vi"("State(s) in (\"\")"=w69) -> ("States Out"=w68:string)  [unwired: 14 in]
      }
      frame "Error Handler" {
        # "Unhandled Error -- Display it"
        # "Handle any errors here.\nYou can also output any states to clean-up after errors occur"
        # "Clear error"
        n28 = call <vilib>:"General Error Handler.vi"("error in (no error)"=w71) -> ()  [unwired: 10 in, 5 out]
        n29 = call <vilib>:"Add State(s) to Queue__jki_lib_state_machine.vi"("State(s) in Front (\"\")"="/* Post Error States", "State(s) in (\"\")"=w75) -> ("States Out"=w74:string)  [unwired: 13 in]
      }
      frame "Exit" {
        # "Do not put any code in this frame.\n(No errors that occur here will be handled.)"
        n30 = call <vilib>:"Add State(s) to Queue__jki_lib_state_machine.vi"("State(s) in (\"\")"=w80) -> ("States Out"=w79:string)  [unwired: 14 in]
      }
      frame "---------- Data ----------" {
        # "Do not put any code in this frame.\n(It is a separator no-op. You can make a copy of this frame to create a new Data frame)"
        n31 = call <vilib>:"Add State(s) to Queue__jki_lib_state_machine.vi"("State(s) in (\"\")"=w84) -> ("States Out"=w83:string)  [unwired: 14 in]
      }
      frame "Data: Initialize" {
        w87 = FALSE  # Mouse Identified
        w88 = T10 {"Area"=0.0, "Number of Holes"=0.0, "Bounding Rect"={"Left"=0.0, "Top"=0.0, "Right"=0.0, "Bottom"=0.0}, "Center of Mass"={"X"=0.0, "Y"=0.0}, "Orientation"=0.0, "Dimensions"={"Width"=0.0, "Height"=0.0}}  # Particle Report
        w89 = T3 refnum  # Processed Diff Image
        (unwired) T11 {"Mouse Image"=refnum, "Mouse Difference Image"=refnum, "Position"={"X"=0, "Y"=0}, "Angle"=0, "Spine Contour"=[], "Outline Contour"=[], "Timestamp"=0, "Height"=0, "Width"=0, "Length"=0, "Area"=0, "Perimeter"=0, "POI Offsets"=[]} ("Mouse Data")
        w90 = T3 refnum  # Processed Background Image
        w91 = T3 refnum  # Occupancy Map
        w92 = T3 refnum  # Processed Image
        w93 = T3 refnum  # Particle Mask
        w94 = 0  # Timestamp
        w101 = 2 items=["Undefined", "Resolution640x480Fps30", "Resolution320x240Fps30", "Resolution80x60Fps30"] ("Depth Format")
        w95 = T3 refnum  # Difference Image
        w102 = T3 refnum  # Raw Image
        w104 = T12 {"Current VI Reference"=refnum, "Close Panel on Exit?"=FALSE}  # Core
        # "Data names and types of shift register data are defined by this bundle."
        # "Initialize the shift-register data, here.\n(data names are defined by what you wire into the bundle function)"
        n32 = call "Kinect Open Baseline Image.vi"() -> ("Background Image Path"=w100:path, "Background Image"=w103:T3)  [unwired: 9 in, 1 out]
        n33 = call "Kinect Create.vi"("Depth Format"=w101) -> ("error out"=w97:errorcluster, "Kinect Acquisition Queue"=w99:refnum<queue>)  [unwired: 9 in]
        n34 = Bundle("Core"=w104, "Background Image"=w103, "Background Image Path"=w100, "Processed Background Image"=w90, "Kinect Acquisition Queue"=w99, "Raw Image"=w102, "Difference Image"=w95, "Processed Image"=w92, "Processed Diff Image"=w89, "Particle Mask"=w93, "Occupancy Map"=w91, "Timestamp"=w94, "Mouse Data"=T5 {"Mouse Image"=refnum, "Mouse Difference Image"=refnum, "Angle"=0, "Spine Contour"=[], "Outline Contour"=[], "Timestamp"=0.0, "Height"=0, "Width"=0, "Length"=0, "Area"=0.0, "POI Offsets"=[], "Frame ID"=0, "Centroid X"=0, "Centroid Y"=0, "Head X"=0, "Head Y"=0, "Tail X"=0, "Tail Y"=0}, "Particle Report"=w88, "Mouse Identified"=w87, "refnum out"=refnum<file> refnum) -> (w105:T9)  [unwired: 1 in]
        n35 = call <vilib>:"Add State(s) to Queue__jki_lib_state_machine.vi"("State(s) in (\"\")"=w107) -> ("States Out"=w106:string)  [unwired: 14 in]
        n36 = Select(t=w97, s=w96, f=w96) -> (s? t:f=w98:errorcluster)
      }
      frame "Data: Allocate Images" {
        w111 = T13 1 items=["Grayscale (U8)", "Grayscale (I16)", "Grayscale (SGL)", "Complex (CSG)", "RGB (U32)", "HSL (U32)", "RGB (U64)", "Grayscale (U16)"] ("Image Type")
        w112 = T13 1 items=["Grayscale (U8)", "Grayscale (I16)", "Grayscale (SGL)", "Complex (CSG)", "RGB (U32)", "HSL (U32)", "RGB (U64)", "Grayscale (U16)"] ("Image Type")
        w125 = T13 2 items=["Grayscale (U8)", "Grayscale (I16)", "Grayscale (SGL)", "Complex (CSG)", "RGB (U32)", "HSL (U32)", "RGB (U64)", "Grayscale (U16)"] ("Image Type")
        w124 = T13 0 items=["Grayscale (U8)", "Grayscale (I16)", "Grayscale (SGL)", "Complex (CSG)", "RGB (U32)", "HSL (U32)", "RGB (U64)", "Grayscale (U16)"] ("Image Type")
        w126 = T13 1 items=["Grayscale (U8)", "Grayscale (I16)", "Grayscale (SGL)", "Complex (CSG)", "RGB (U32)", "HSL (U32)", "RGB (U64)", "Grayscale (U16)"] ("Image Type")
        w127 = T13 1 items=["Grayscale (U8)", "Grayscale (I16)", "Grayscale (SGL)", "Complex (CSG)", "RGB (U32)", "HSL (U32)", "RGB (U64)", "Grayscale (U16)"] ("Image Type")
        w131 = T13 1 items=["Grayscale (U8)", "Grayscale (I16)", "Grayscale (SGL)", "Complex (CSG)", "RGB (U32)", "HSL (U32)", "RGB (U64)", "Grayscale (U16)"] ("Image Type")
        w130 = T13 1 items=["Grayscale (U8)", "Grayscale (I16)", "Grayscale (SGL)", "Complex (CSG)", "RGB (U32)", "HSL (U32)", "RGB (U64)", "Grayscale (U16)"] ("Image Type")
        n37 = call "IMAQ Create"("Image Name"="Raw Image", "Image Type"=w130) -> ("New Image"=w122:T3)  [unwired: 3 in, 1 out]
        n38 = call "IMAQ Create"("Image Name"="Processed Image", "Image Type"=w127) -> ("New Image"=w119:T3)  [unwired: 3 in, 1 out]
        n39 = call "IMAQ Create"("Image Name"="Particle Mask", "Image Type"=w124) -> ("New Image"=w116:T3)  [unwired: 3 in, 1 out]
        n40 = call "IMAQ Create"("Image Name"="Mouse Image", "Image Type"=w112) -> ("New Image"=w110:T3)  [unwired: 3 in, 1 out]
        n41 = call "IMAQ Create"("Image Name"="Difference Image", "Image Type"=w131) -> ("New Image"=w120:T3)  [unwired: 3 in, 1 out]
        n42 = call "IMAQ Create"("Image Name"="Processed Diff Image", "Image Type"=w126) -> ("New Image"=w117:T3)  [unwired: 3 in, 1 out]
        n43 = call "IMAQ Create"("Image Name"="Occupancy Map", "Image Type"=w125) -> ("New Image"=w114:T3)  [unwired: 3 in, 1 out]
        n44 = call "IMAQ Create"("Image Name"="Mouse Difference Image", "Image Type"=w111) -> ("New Image"=w109:T3)  [unwired: 3 in, 1 out]
        n45 = Bundle By Name(cluster=w133, "Raw Image"=w122, "Difference Image"=w120, "Processed Image"=w119, "Processed Diff Image"=w117, "Particle Mask"=w116, "Occupancy Map"=w114, "Mouse Data.Mouse Image"=w110, "Mouse Data.Mouse Difference Image"=w109) -> (w132:T9)
        n46 = call <vilib>:"Add State(s) to Queue__jki_lib_state_machine.vi"("State(s) in (\"\")"=w136) -> ("States Out"=w135:string)  [unwired: 14 in]
      }
      frame "Data: Cleanup" {
        # "Cleanup any data and references, here.\n(this is called automatically, by the Macro: Exit)"
        n47 = Unbundle By Name(w141) -> ("Core.Current VI Reference"=w143:refnum<vi>, "Kinect Acquisition Queue"=w137:refnum<queue>)
        n48 = Release Queue(queue=w137, error in (no error)=w138) -> (error out=w139:errorcluster)  [unwired: 1 in, 2 out]
        n49 = call "Kinect Destroy.vi"("error in"=w139) -> ("error out"=w140:errorcluster)  [unwired: 10 in]
        n50 = Close Reference(reference=w143, error in (no error)=w140) -> (error out=w142:errorcluster)
        n51 = call <vilib>:"Add State(s) to Queue__jki_lib_state_machine.vi"("State(s) in (\"\")"=w145) -> ("States Out"=w144:string)  [unwired: 14 in]
      }
      frame "---------- UI ----------" {
        # "Do not put any code in this frame.\n(It is a separator no-op. You can make a copy of this frame to create a new UI frame)"
        n52 = call <vilib>:"Add State(s) to Queue__jki_lib_state_machine.vi"("State(s) in (\"\")"=w149) -> ("States Out"=w148:string)  [unwired: 14 in]
      }
      frame "UI: Initialize" {
        # "Initialize the User Interface, here.\n(this is called automatically, by the Macro: Init)"
        n53 = call <vilib>:"Add State(s) to Queue__jki_lib_state_machine.vi"("State(s) in (\"\")"=w153) -> ("States Out"=w152:string)  [unwired: 14 in]
      }
      frame "UI: Cursor Set" {
        # "Argument"
        # "Set and Unset Cursor Busy.\n(Usage: \"UI: Cursor Set >> Busy|Idle\")"
        n54 = case shown="\"Idle\", Default" w154 {
          tunnel: w156 -> [w161 w163]
          tunnel: [w160 w162] -> w155
          frame "Idle", Default {
            n55 = call <vilib>:"Unset Busy.vi"("error in (no error)"=w161) -> ("error out"=w160:errorcluster)  [unwired: 10 in]
          }
          frame "Busy" {
            n56 = call <vilib>:"Set Busy.vi"("error in (no error)"=w163) -> ("error out"=w162:errorcluster)  [unwired: 9 in, 1 out]
          }
        }
        n57 = call <vilib>:"Add State(s) to Queue__jki_lib_state_machine.vi"("State(s) in (\"\")"=w159) -> ("States Out"=w158:string)  [unwired: 14 in]
      }
      frame "UI: Front Panel State" {
        # "Argument"
        # "Set Front Panel Open or Closed\n(Usage: \"UI: Front Panel State >> Open|Close\")"
        n58 = Unbundle By Name(w166) -> ("Core.Current VI Reference"=w165:refnum<vi>)
        n59 = case shown="\"Open\", Default" w164 {
          tunnel: w168 -> [w174 w187]
          tunnel: [w176 w188] -> w167
          tunnel: w165 -> [w175 w185]
          frame "Open", Default {
            n60 = property class="VI"(reference=w175, error in=w174) -> (reference out=w172:refnum<vi>, error out=w173:errorcluster, "Front Panel.Open"=w171:bool)
            n61 = case shown="True" w171 {
              tunnel: [w179 w182] -> w176
              tunnel: w173 -> [w178 w182]
              tunnel: w172 -> [w177 _]
              frame False {
                n62 = invoke class="VI" method="FP.Open"(reference=w177, error in=w178, "Activate"=TRUE, "State"=T6."Standard") -> (error out=w179:errorcluster)  [unwired: 1 in, 4 out]
              }
              frame True {
              }
            }
          }
          frame "Close" {
            n63 = property class="VI"(reference=w185, error in=w187) -> (reference out=w184:refnum<vi>, error out=w186:errorcluster, "Front Panel.Open"=w183:bool)
            n64 = case shown="True" w183 {
              tunnel: [w189 w192] -> w188
              tunnel: w186 -> [w189 w191]
              tunnel: w184 -> [_ w190]
              frame False {
              }
              frame True {
                n65 = invoke class="VI" method="FP.Close"(reference=w190, error in=w191) -> (error out=w192:errorcluster)  [unwired: 1 in, 2 out]
              }
            }
          }
        }
        n66 = call <vilib>:"Add State(s) to Queue__jki_lib_state_machine.vi"("State(s) in (\"\")"=w170) -> ("States Out"=w169:string)  [unwired: 14 in]
      }
      frame "---------- Macro ----------" {
        # "Do not put any code in this frame.\n(It is a separator no-op. You can make a copy of this frame to create a new Macro frame)"
        n67 = call <vilib>:"Add State(s) to Queue__jki_lib_state_machine.vi"("State(s) in (\"\")"=w196) -> ("States Out"=w195:string)  [unwired: 14 in]
      }
      frame "Macro: Initialize" {
        w197 = "Data: Initialize\nData: Allocate Images\nInitialize Core Data\nUI: Initialize\nUI: Front Panel State >> Open\nIO: Open File\nImage: Process Background"  # Data: Initialize Data: Allocate Images Initialize Core Data UI: Initialize UI: Front Panel State >> Open IO: Open File Image: Process Background
        # "Initialization Macro\n(This is called once, when the VI starts)"
        n68 = call <vilib>:"Add State(s) to Queue__jki_lib_state_machine.vi"("State(s) in Front (\"\")"=w197, "State(s) in (\"\")"=w201) -> ("States Out"=w200:string)  [unwired: 13 in]
      }
      frame "Macro: Exit" {
        # "Exit Macro\n(This is called once, when the VI exits)"
        n69 = Unbundle By Name(w208) -> ("Core.Close Panel on Exit?"=w207:bool)
        n70 = Select(t="UI: Front Panel State >> Close", s=w207, f="") -> (s? t:f=w204:string)
        n71 = call <vilib>:"Add State(s) to Queue__jki_lib_state_machine.vi"("State(s) in (\"\")"=w204, "State(s) at Back (\"\")"="Data: Cleanup\nExit") -> ("States Out"=w202:string)  [unwired: 13 in]
        n72 = call <vilib>:"Add State(s) to Queue__jki_lib_state_machine.vi"("State(s) in Front (\"\")"=w202, "State(s) in (\"\")"=w211) -> ("States Out"=w210:string)  [unwired: 13 in]
      }
      frame "---------- Control ----------" {
        # "Template Separator\n(You can make a copy of, or modify, this frame)"
        n73 = call <vilib>:"Add State(s) to Queue__jki_lib_state_machine.vi"("State(s) in (\"\")"=w215) -> ("States Out"=w214:string)  [unwired: 14 in]
      }
      frame "Control: Idle" {
        n74 = call <vilib>:"Add State(s) to Queue__jki_lib_state_machine.vi"("State(s) in Front (\"\")"="Image: Acquire\nImage: Preprocess\nImage: Find Particles\nImage: Correct Orientation\nImage: Extract Particles\nImage: Analyze Particles\n Image: Find Head vs Tail\nImage: Update Heat Map\nImage: Display" ("State(s) in Front (\"\")"), "State(s) in (\"\")"=w220) -> ("States Out"=w219:string)  [unwired: 13 in]
      }
      frame "Control: Playback" {
        n75 = call <vilib>:"Add State(s) to Queue__jki_lib_state_machine.vi"("State(s) in Front (\"\")"="Image: Acquire From File\nImage: Preprocess From File\nImage: Find Particles\nImage: Correct Orientation\nImage: Extract Particles\nImage: Analyze Particles\nImage: Align On Butt\n Image: Find Head vs Tail\nImage: Update Heat Map\nImage: Display\nIO: Write Frame" ("State(s) in Front (\"\")"), "State(s) in (\"\")"=w225) -> ("States Out"=w224:string)  [unwired: 13 in]
      }
      frame "Control: Record" {
        n76 = call <vilib>:"Add State(s) to Queue__jki_lib_state_machine.vi"("State(s) in Front (\"\")"="Image: Acquire\nImage: Preprocess\nImage: Find Particles\nImage: Update Heat Map\n// IO: Save Frame\nImage: Display" ("State(s) in Front (\"\")"), "State(s) in (\"\")"=w230) -> ("States Out"=w229:string)  [unwired: 13 in]
      }
      frame "Control: Mouse Not Found" {
        # "We hijack the whole control flow,\nhitting us back to the idle state.\nIf we don't have a mouse, then we\ngot nothing to do, really."
        n77 = Bundle By Name(cluster=w234, "Mouse Identified"=FALSE) -> (w233:T9)
        n78 = call <vilib>:"Add State(s) to Queue__jki_lib_state_machine.vi"("State(s) in (\"\")"="Image: Display" ("State(s) in (\"\")")) -> ("States Out"=w236:string)  [unwired: 14 in]
      }
      frame "---------- Image ----------" {
        # "Template Separator\n(You can make a copy of, or modify, this frame)"
        n79 = call <vilib>:"Add State(s) to Queue__jki_lib_state_machine.vi"("State(s) in (\"\")"=w240) -> ("States Out"=w239:string)  [unwired: 14 in]
      }
      frame "Image: Acquire" {
        # "The Kinect provides raw Int16 data to us\nvia a .NET callback. We throw the data into\nthe queue above in the callback,\nand then digest it here, reshape it, and\ncreate an image out of it.\nWe also store the previous image, and create\na \"difference image\", which tells us about\nregions of movement."
        n80 = Unbundle By Name(w249) -> ("Kinect Acquisition Queue"=w250:refnum<queue>, "Mouse Data.Frame ID"=w242:i16)
        n81 = Increment(x=w242) -> (x+1=w241:i16)
        n82 = call "Kinect Acquire.vi"("error in"=w244, "Queue in"=w250) -> ("error out"=w243:errorcluster, "Timestamp"=w245:i32, "Difference\nImage"=w246:T3, "Image Out"=w247:T3)  [unwired: 6 in]
        n83 = Bundle By Name(cluster=w249, "Raw Image"=w247, "Difference Image"=w246, "Timestamp"=w245, "Mouse Data.Frame ID"=w241) -> (w248:T9)
        n84 = call <vilib>:"Add State(s) to Queue__jki_lib_state_machine.vi"("State(s) in (\"\")"=w252) -> ("States Out"=w251:string)  [unwired: 14 in]
      }
      frame "Image: Acquire From File" {
        # "NOTE: This will only work once per VI call.\nShould be spruced up a bit in the fyutchah."
        n85 = Wait (ms)(milliseconds to wait="Milliseconds to wait between frames") -> ()  [unwired: 1 out]
        n86 = call "Kinect Acquire From File.vi"("error in"=w264, "Path to Folder\nContaining TIFF Images"="Path to Folder\nContaining TIFF Images") -> ("error out"=w263:errorcluster, "Out of Frames?"=w262:bool, "Diff Image Out"=w265:T3, "Image Out"=w266:T3)  [unwired: 6 in]
        n87 = Unbundle By Name(w260) -> ("Processed Background Image"=w259:T3, "Mouse Data.Frame ID"=w255:i16)
        n88 = call "Get Unix Time.vi"() -> ("Unix time"=w253:dbl)  [unwired: 10 in, 1 out]
        n89 = Increment(x=w255) -> (x+1=w254:i16)
        n90 = call "IMAQ FillImage"("Pixel Value (U8, U16, I16, Float)"=sgl 0.0, "Image"=w259) -> ("Image Out"=w257:T3)  [unwired: 8 in, 1 out]
        n91 = Bundle By Name(cluster=w260, "Raw Image"=w266, "Difference Image"=w265, "Mouse Data.Timestamp"=w253, "Processed Background Image"=w257, "Mouse Data.Frame ID"=w254) -> (w268:T9)
        n92 = case shown="True" w262 {
          tunnel: ["" ("State(s) in Front (\"\")") "IO: Close File\nMacro: Exit" ("State(s) in Front (\"\")")] -> w261
          frame False {
          }
          frame True {
          }
        }
        n93 = call <vilib>:"Add State(s) to Queue__jki_lib_state_machine.vi"("State(s) in Front (\"\")"=w261, "State(s) in (\"\")"=w270) -> ("States Out"=w269:string)  [unwired: 13 in]
      }
      frame "Image: Preprocess" {
        w291 = 2.0  # Standard Deviation
        # "The raw image off the Kinect requires significant\nprocessing to be useful for mouse tracking.\nNamely, we have to subtract off the background,\nperform median filtering, and then thresholding.\nThen, we apply a pretty heavy blur for good measure."
        n94 = Unbundle By Name(w283) -> ("Processed Image"=w289:T3, "Processed Background Image"=w286:T3, "Raw Image"=w285:T3)
        n95 = Unbundle By Name(w283) -> ("Difference Image"=w274:T3)
        n96 = call "Kinect Extract Background 2.vi"("Background Image In"=w286, "Depth Image In"=w285, "Median Filter Size"="Median Filter Size", "Divisor"="Divisor", "Distance to Camera Visible"="Distance to Camera Visible", "Post Proc Bounds"="Post Extraction Limit", "error in"=w279) -> ("Processed Image Out"=w288:T3, "error out"=w287:errorcluster)  [unwired: 19 in]
        n97 = call "Kinect Process Image.vi"("Depth Image In"=w274, "Distance to Camera Visible"="Distance to Camera Visible 2", "Median Filter Size"="Median Filter Size 2", "Divisor"="Divisor 2") -> ("Image Dst Out"=w273:T3)  [unwired: 10 in, 1 out]
        n98 = call "Gaussian Blur.vi"("Image"=w288, "Image Dst"=w289, "Kernel Size"="Gaussian Blur Kernel Size", "Standard Deviation"=w291, "error in"=w287) -> ("Image Out"=w290:T3, "error out"=w280:errorcluster)  [unwired: 9 in]
        n99 = Bundle By Name(cluster=w283, "Processed Image"=w290, "Processed Diff Image"=w273) -> (w293:T9)
        n100 = call <vilib>:"Add State(s) to Queue__jki_lib_state_machine.vi"("State(s) in (\"\")"=w295) -> ("States Out"=w294:string)  [unwired: 14 in]
      }
      frame "Image: Preprocess From File" {
        w307 = 2.0  # Standard Deviation
        n101 = Unbundle By Name(w304) -> ("Processed Image"=w305:T3, "Raw Image"=w296:T3)  [unwired: 1 out]
        n102 = Unbundle By Name(w304) -> ("Difference Image"=w299:T3)
        n103 = call "Kinect Process Image.vi"("Depth Image In"=w299, "Distance to Camera Visible"="Distance to Camera Visible 3", "Median Filter Size"="Median Filter Size (From File)", "Divisor"="Divisor For Filter (From File)") -> ("Image Dst Out"=w298:T3)  [unwired: 10 in, 1 out]
        n104 = call "Gaussian Blur.vi"("Image"=w296, "Image Dst"=w305, "Kernel Size"="Gaussian Blur Kernel Size (From File)", "Standard Deviation"=w307, "error in"=w297) -> ("Image Out"=w306:T3, "error out"=w303:errorcluster)  [unwired: 9 in]
        n105 = Bundle By Name(cluster=w304, "Processed Image"=w306, "Processed Diff Image"=w298) -> (w309:T9)
        n106 = call <vilib>:"Add State(s) to Queue__jki_lib_state_machine.vi"("State(s) in (\"\")"=w311) -> ("States Out"=w310:string)  [unwired: 14 in]
      }
      frame "Image: Find Particles" {
        # "If we don't find any particles, we gotta jet the heck out"
        # "Selection Range is the pixel distances within which we allow particles to be found\nSelection Parameters is an array of different particle properties we use to pick particles\nthat we think would be reasonable. Mostly, I just select for reasonable areas. Above 300px^2, but\nless than 1500px^2."
        n107 = Unbundle By Name(w320) -> ("Processed Image"=w326:T3)
        n108 = call "Kinect Find Blobs.vi"("Image Src"=w326, "Selection Values"="Selection Parameters 2", "Number of Erosion"="Number of Erosion 2", "Range"="Selection Range 2", "error in"=w323) -> ("Masked Image Out"=w317:T3, "Particle Reports (Pixels)"=w316:T14, "error out"=w322:errorcluster)  [unwired: 7 in, 1 out]
        n109 = Index Array(array=w316, index=0) -> (element=w319:T10)
        n110 = Array Size(array=w316) -> (size(s)=w315:i32)
        n111 = Less?(x=w315, y=1) -> (x < y?=w313:bool)
        n112 = Bundle By Name(cluster=w320, "Particle Mask"=w317, "Particle Report"=w319) -> (w318:T9)
        n113 = case shown="False" w313 {
          tunnel: ["" "Control: Mouse Not Found"] -> w312
          frame False {
          }
          frame True {
          }
        }
        n114 = call <vilib>:"Add State(s) to Queue__jki_lib_state_machine.vi"("State(s) in Front (\"\")"=w312, "State(s) in (\"\")"=w329) -> ("States Out"=w328:string)  [unwired: 13 in]
      }
      frame "Image: Correct Orientation" {
        w342 = 120
        # "If an absolute angle difference is greater than 120, \nkeep flipping it around 180 degrees until it's less than 120"
        n115 = Unbundle By Name(w337) -> ("Particle Report.Orientation"=w332:dbl)
        n116 = Negate(x=w342) -> (-x=w344:i32)
        n117 = feedback #1(w332) -> (w338:dbl)
        n118 = Subtract(x=w332, y=w338) -> (x-y=w345:dbl)
        n119 = Subtract(x=w332, y=w338) -> (x-y=w343:dbl)
        n120 = Greater Or Equal?(x=w343, y=w342) -> (x >= y?=w341:bool)
        n121 = Less Or Equal?(x=w345, y=w344) -> (x <= y?=w339:bool)
        n122 = Or(x=w339, y=w341) -> (x .or. y?=w340:bool)
        n123 = case shown="True" w340 {
          tunnel: [w354 w360] -> w335
          tunnel: w342 -> [_ w359]
          tunnel: w332 -> [w354 w358]
          tunnel: w338 -> [_ w357]
          tunnel: w339 -> [_ w356]
          frame False {
          }
          frame True {
            n124 = case shown="True" w356 {
              tunnel: [-180.0 ("y") 180.0 ("y")] -> w355
              frame False {
              }
              frame True {
              }
            }
            n125 = while {
              tunnel: w357 -> [w368]
              tunnel: w359 -> [w365]
              tunnel: w355 -> [w363]
              shift-right: [w369] -> w360
              shift-left: w358 -> [w370]
              stop <- w364 continue-if-true
              n126 = Add(x=w370, y=w363) -> (x+y=w369:dbl)
              n127 = Subtract(x=w369, y=w368) -> (x-y=w367:dbl)
              n128 = Absolute Value(x=w367) -> (abs(x)=w366:dbl)
              n129 = Greater?(x=w366, y=w365) -> (0:w364:bool)
            }
          }
        }
        n130 = case shown="True" "Flip?" {
          tunnel: [w349 w352] -> w334
          tunnel: w335 -> [w349 w353]
          frame False {
          }
          frame True {
            n131 = Add(x=w353, y=180.0) -> (x+y=w352:dbl)
            n132 = local write "Flip?"(FALSE ("Flip?")) -> ()
          }
        }
        n133 = feedback-in #1(w334) -> ()
        n134 = Bundle By Name(cluster=w337, "Mouse Data.Angle"=w334, "Particle Report.Orientation"=w334) -> (w336:T9)
        n135 = call <vilib>:"Add State(s) to Queue__jki_lib_state_machine.vi"("State(s) in (\"\")"=w348) -> ("States Out"=w347:string)  [unwired: 14 in]
      }
      frame "Image: Extract Particles" {
        # "Once we have a good preprocessed image where only the animals\nare visible in the scene, we can threshold the image, creating a \nbinary mask (with some speckle noise). We then find contiguous\nlight regions in the binary image with an area within a specified range,\nand then remove all other light regions that don't fit the criteria."
        # "Selection Range is the pixel distances within which we allow particles to be found\nSelection Parameters is an array of different particle properties we use to pick particles\nthat we think would be reasonable. Mostly, I just select for reasonable areas. Above 300px^2, but\nless than 1500px^2."
        n136 = Unbundle By Name(w371) -> ("Processed Diff Image"=w375:T3, "Mouse Data.Mouse Difference Image"=w374:T3)
        n137 = Unbundle By Name(w371) -> ("Particle Mask"=w379:T3, "Particle Report"=w378:T10)
        n138 = Unbundle By Name(w371) -> ("Processed Image"=w377:T3, "Mouse Data.Mouse Image"=w376:T3)
        n139 = call "Kinect Extract Mouse 2.vi"("Image Src"=w375, "Image Mask"=w379, "Cropped Image Src"=w374, "Particle Report"=w378, "error in (no error)"=w384, "Width"="Width", "Height"="Height") -> ("Extracted Particle"=w372:T3, "error out"=w383:errorcluster)  [unwired: 11 in]
        n140 = call "Kinect Extract Mouse 2.vi"("Image Src"=w377, "Image Mask"=w379, "Cropped Image Src"=w376, "Particle Report"=w378, "error in (no error)"=w383, "Width"="Width", "Height"="Height") -> ("Extracted Particle"=w373:T3, "error out"=w382:errorcluster)  [unwired: 11 in]
        n141 = Bundle By Name(cluster=w371, "Mouse Data.Mouse Image"=w373, "Mouse Data.Mouse Difference Image"=w372) -> (w385:T9)
        n142 = call <vilib>:"Add State(s) to Queue__jki_lib_state_machine.vi"("State(s) in (\"\")"=w387) -> ("States Out"=w386:string)  [unwired: 14 in]
      }
      frame "Image: Find Head vs Tail" {
        # "Essentially, if we find a head or a tail\nin the image, that means we can really\nstart tracking the mouse. Before that point,\nwe really don't have enough information\nto save out data to disk."
        # "Find the difference of standard deviation \nbetween left vs right side of the image"
        n143 = Unbundle By Name(w389) -> ("Mouse Data.Mouse Difference Image"=w397:T3)
        n144 = feedback #2() -> (w392:bool)  [unwired: 1 in]
        n145 = call "Identify Head vs Tail in Difference Image.vi"("History Length \nfor Head v Tail Determination"="History Length \nfor Head v Tail Determination", "Reset?"=w392, "Diff Image In"=w397) -> ("Significant?"=w391:bool, "Facing Left?"=w390:bool)  [unwired: 7 in]
        n146 = case shown="True" w391 {
          tunnel: w390 -> [_ w411]
          tunnel: [w404 w410] -> w396
          tunnel: ["" ("String") w409] -> w395
          tunnel: [FALSE ("Flip?") w408] -> w393
          tunnel: w389 -> [w401 w407]
          tunnel: [w401 w406] -> w388
          frame False {
            # "No significant bead on which end is the head or tail.\nWe won't do anything."
            n147 = local read "Movement \nDecision"() -> (w404:string)
          }
          frame True {
            # "We've got a directionality!"
            n148 = case shown="False" w411 {
              tunnel: [">" "<"] -> w410
              tunnel: ["" ("String") "Image: Correct Orientation\nImage: Extract Particles\nImage: Find Head Vs Tail"] -> w409
              tunnel: [FALSE ("Flip?") w415] -> w408
              frame False {
                # "Head's on the right. All's well."
              }
              frame True {
                w415 = TRUE ("Flip?")
                # "Aight, the head's on the left. We want it on the right.\nFix it."
                n149 = local write "Flip?"(w415) -> ()
              }
            }
            n150 = Bundle By Name(cluster=w407, "Mouse Identified"=TRUE) -> (w406:T9)
          }
        }
        "Movement \nDecision" <- w396
        n151 = feedback-in #2(w393) -> ()
        n152 = call <vilib>:"Add State(s) to Queue__jki_lib_state_machine.vi"("State(s) in Front (\"\")"=w395, "State(s) in (\"\")"=w400) -> ("States Out"=w399:string)  [unwired: 13 in]
      }
      frame "Image: Align On Butt" {
        # "We want the butt of the mouse at a fixed position between frames."
        n153 = Unbundle By Name(w426) -> ("Mouse Data.Spine Contour"=w422:i32[], "Mouse Data.Mouse Image"=w423:T3, "Mouse Data.Mouse Difference Image"=w419:T3)
        n154 = call "Kinect Offset Image To Base Of Contour.vi"("Image In"=w423, "Spine Contour"=w422, "Butt Position (pixels from left of image)"="Butt Position (pixels from left of image)", "Butt Threshold"="Butt Threshold") -> ("Image Out"=w427:T3)  [unwired: 11 in]
        n155 = call "Kinect Offset Image To Base Of Contour.vi"("Image In"=w419, "Spine Contour"=w422, "Butt Position (pixels from left of image)"="Butt Position (pixels from left of image)", "Butt Threshold"="Butt Threshold") -> ("Image Out"=w418:T3)  [unwired: 11 in]
        n156 = Bundle By Name(cluster=w426, "Mouse Data.Mouse Image"=w427, "Mouse Data.Mouse Difference Image"=w418) -> (w425:T9)
        n157 = call <vilib>:"Add State(s) to Queue__jki_lib_state_machine.vi"("State(s) in Front (\"\")"="Image: Analyze Particles" ("State(s) in Front (\"\")"), "State(s) in (\"\")"=w430) -> ("States Out"=w429:string)  [unwired: 13 in]
      }
      frame "Image: Analyze Particles" {
        n158 = Unbundle By Name(w452) -> ("Particle Mask"=w450:T3, "Mouse Data.Mouse Image"=w438:T3, "Mouse Data.Angle"=w432:i32, "Mouse Data.Timestamp"=w431:dbl)
        n159 = local read "Butt Threshold"() -> (w437:dbl)
        n160 = call "Kinect Analyze Particle.vi"("Particle Mask In"=w450, "Extracted Mouse Image"=w438, "Height Threshold"=w437, "Mouse Orientation"=w432, "error in"=w449) -> ("Mouse Data"=w447:T5, "error out"=w448:errorcluster)  [unwired: 9 in]
        n161 = Unbundle By Name(w447) -> ("Head X"=w436:i32, "Head Y"=w435:i32, "Tail X"=w434:i32, "Tail Y"=w433:i32, "Centroid X"=w446:i32, "Centroid Y"=w445:i32, "Area"=w444:sgl, "Spine Contour"=w443:i32[], "Outline Contour"=w442:i32[][], "Height"=w441:i32, "Width"=w440:i32, "Length"=w439:i32)
        n162 = Bundle By Name(cluster=w452, "Mouse Data.Head X"=w436, "Mouse Data.Head Y"=w435, "Mouse Data.Tail X"=w434, "Mouse Data.Tail Y"=w433, "Mouse Data.Centroid X"=w446, "Mouse Data.Centroid Y"=w445, "Mouse Data.Area"=w444, "Mouse Data.Spine Contour"=w443, "Mouse Data.Outline Contour"=w442, "Mouse Data.Height"=w441, "Mouse Data.Width"=w440, "Mouse Data.Length"=w439, "Timestamp"=w431) -> (w451:T9)
        n163 = call <vilib>:"Add State(s) to Queue__jki_lib_state_machine.vi"("State(s) in (\"\")"=w454) -> ("States Out"=w453:string)  [unwired: 14 in]
      }
      frame "Image: Update Heat Map" {
        # "We keep track of an occupancy map of the animal. This will show us, in a \"heat map\" fashion,\nhow much time the animal has spent throughout the experimental area."
        n164 = Unbundle By Name(w462) -> ("Particle Mask"=w460:T3, "Occupancy Map"=w459:T3)
        n165 = Empty String/Path?(string/path=w459) -> ()  [unwired: 1 out]
        n166 = case shown="False" FALSE {
          tunnel: [w472 w485] -> w458
          tunnel: w460 -> [w476 w484]
          tunnel: w459 -> [w473 _]
          tunnel: [w467 w483] -> w457
          tunnel: w456 -> [w466 w480]
          frame False {
            w474 = T13 2 items=["Grayscale (U8)", "Grayscale (I16)", "Grayscale (SGL)", "Complex (CSG)", "RGB (U32)", "HSL (U32)", "RGB (U64)", "Grayscale (U16)"] ("Image Type")
            w477 = T13 2 items=["Grayscale (U8)", "Grayscale (I16)", "Grayscale (SGL)", "Complex (CSG)", "RGB (U32)", "HSL (U32)", "RGB (U64)", "Grayscale (U16)"] ("Image Type")
            # "Add the particle mask (where there are 1's where there's an animal\nand 0's where there aren't) to the occupancy map"
            n167 = call "IMAQ Create"("Image Name"="Heat Tmp", "Image Type"=w474, "error in (no error)"=w466) -> ("New Image"=w465:T3, "error out"=w470:errorcluster)  [unwired: 2 in]
            n168 = call "IMAQ Cast Image"("Image Type"=w477, "error in (no error)"=w470, "Image Dst"=w465, "Image Src"=w476) -> ("error out"=w471:errorcluster, "Image Dst Out"=w468:T3)  [unwired: 6 in]
            n169 = call "IMAQ Add"("Image Src A"=w468, "Image Dst"=w473, "Image Src B"=w473, "error in (no error)"=w471) -> ("Image Dst Out"=w472:T3, "error out"=w469:errorcluster)  [unwired: 3 in]
            n170 = call "IMAQ Dispose"("Image"=w465, "error in (no error)"=w469) -> ("error out"=w467:errorcluster)  [unwired: 4 in]
          }
          frame True {
            w481 = T13 2 items=["Grayscale (U8)", "Grayscale (I16)", "Grayscale (SGL)", "Complex (CSG)", "RGB (U32)", "HSL (U32)", "RGB (U64)", "Grayscale (U16)"] ("Image Type")
            w486 = T13 2 items=["Grayscale (U8)", "Grayscale (I16)", "Grayscale (SGL)", "Complex (CSG)", "RGB (U32)", "HSL (U32)", "RGB (U64)", "Grayscale (U16)"] ("Image Type")
            # "If the occupancy map hasn't been created, first create it as an image of floats."
            n171 = call "IMAQ Create"("Image Name"="Occupancy Map", "Image Type"=w481, "error in (no error)"=w480) -> ("New Image"=w478:T3, "error out"=w479:errorcluster)  [unwired: 2 in]
            n172 = call "IMAQ Cast Image"("Image Type"=w486, "error in (no error)"=w479, "Image Dst"=w478, "Image Src"=w484) -> ("error out"=w483:errorcluster, "Image Dst Out"=w485:T3)  [unwired: 6 in]
          }
        }
        n173 = Bundle By Name(cluster=w462, "Occupancy Map"=w458) -> (w461:T9)
        n174 = call <vilib>:"Add State(s) to Queue__jki_lib_state_machine.vi"("State(s) in (\"\")"=w464) -> ("States Out"=w463:string)  [unwired: 14 in]
      }
      frame "Image: Display" {
        n175 = Unbundle By Name(w499) -> ("Processed Image"=w489:T3, "Processed Diff Image"=→"Diff Image":T3, "Particle Mask"=→"Mask":T3, "Occupancy Map"=→"Heat Map":T3, "Mouse Data.Mouse Image"=→"Extracted Image":T3, "Mouse Data.Mouse Difference Image"=→"Extracted Diff Image":T3, "Mouse Data.Spine Contour"=→"Spine Contour":i32[])
        n176 = Unbundle By Name(w499) -> ("Mouse Data.Head X"=w494:i32, "Mouse Data.Head Y"=w493:i32, "Mouse Data.Centroid X"=w496:i32, "Mouse Data.Centroid Y"=w495:i32, "Mouse Data.Tail X"=w498:i32, "Mouse Data.Tail Y"=w497:i32)
        n177 = Bundle("Head X"=w494, "Head Y"=w493) -> (w492:cluster{"Head X":i32, "Head Y":i32})  [unwired: 1 in]
        n178 = Bundle("Centroid X"=w496, "Centroid Y"=w495) -> (w490:cluster{"Centroid X":i32, "Centroid Y":i32})  [unwired: 1 in]
        n179 = Bundle("Tail X"=w498, "Tail Y"=w497) -> (w491:cluster{"Tail X":i32, "Tail Y":i32})  [unwired: 1 in]
        n180 = Build Array(w492, w490, w491) -> (w488:cluster{"Tail X":i32, "Tail Y":i32}[])
        n181 = call <vilib>:"Add State(s) to Queue__jki_lib_state_machine.vi"("State(s) in (\"\")"=w508) -> ("States Out"=w507:string)  [unwired: 14 in]
        n182 = call "IMAQ Overlay Multiple Lines 2"("Image"=w489, "Line End Points"=w488) -> ("Image Out"=→"Raw Image":T3)  [unwired: 12 in, 1 out]
      }
      frame "Image: Process Background" {
        w517 = T13 1 items=["Grayscale (U8)", "Grayscale (I16)", "Grayscale (SGL)", "Complex (CSG)", "RGB (U32)", "HSL (U32)", "RGB (U64)", "Grayscale (U16)"] ("Image Type")
        n183 = Unbundle By Name(w515) -> ("Background Image"=w512:T3)
        n184 = call "IMAQ Create"("Image Name"="Processed Background Image", "Image Type"=w517) -> ("New Image"=w516:T3)  [unwired: 3 in, 1 out]
        n185 = call "IMAQ Copy"("Image Dst"=w516, "Image Src"=w512) -> ("Image Dst Out"=w519:T3)  [unwired: 4 in, 1 out]
        n186 = local read "Distance to Camera Visible"() -> (w510:cluster{dbl, dbl})
        n187 = local read "Median Filter Size"() -> (w511:i32)
        n188 = local read "Divisor"() -> (w509:sgl)
        n189 = call "Kinect Process Image.vi"("Depth Image In"=w519, "Distance to Camera Visible"=w510, "Median Filter Size"=w511, "Divisor"=w509) -> ("Image Dst Out"=w513:T3)  [unwired: 10 in, 1 out]
        n190 = Bundle By Name(cluster=w515, "Processed Background Image"=w513) -> (w514:T9)
        n191 = call <vilib>:"Add State(s) to Queue__jki_lib_state_machine.vi"("State(s) in (\"\")"=w522) -> ("States Out"=w521:string)  [unwired: 14 in]
      }
      frame "Image: Acquire Background" {
        n192 = Unbundle By Name(w533) -> ("Background Image Path"=w527:path, "Kinect Acquisition Queue"=w528:refnum<queue>)
        n193 = for {
          N: "Number of Frames To Average\nfor Background Image" -> [_]
          tunnel: w528 -> [w543]
          shift-right: [w536] -> w524
          shift-left: w529 -> [w542]
          shift-right: [w537] -> w526
          shift-left: _ -> [w538]
          n194 = call "Kinect Acquire.vi"("error in"=w542, "Queue in"=w543) -> ("error out"=w540:errorcluster, "Image Out"=w539:T3)  [unwired: 6 in, 2 out]
          n195 = call "IMAQ Compare"("Operator"=T7."Max", "error in (no error)"=w540, "Image Src B"=w538, "Image Src A"=w539) -> ("error out"=w536:errorcluster, "Image Dst Out"=w537:T3)  [unwired: 6 in]
        }
        n196 = call "Kinect Save Baseline Image.vi"("error in (no error)"=w524, "Baseline Image Path"=w527, "Baseline Image"=w526) -> ("error out"=w523:errorcluster, "Baseline Image Out"=w525:T3)  [unwired: 7 in]
        n197 = Bundle By Name(cluster=w533, "Background Image"=w525) -> (w532:T9)
        n198 = call <vilib>:"Add State(s) to Queue__jki_lib_state_machine.vi"("State(s) in Front (\"\")"="Image: Process Background" ("State(s) in Front (\"\")"), "State(s) in (\"\")"=w535) -> ("States Out"=w534:string)  [unwired: 13 in]
      }
      frame "---------- IO ----------" {
        # "Template Separator\n(You can make a copy of, or modify, this frame)"
        n199 = call <vilib>:"Add State(s) to Queue__jki_lib_state_machine.vi"("State(s) in (\"\")"=w547) -> ("States Out"=w546:string)  [unwired: 14 in]
      }
      frame "IO: Open File" {
        n200 = Open/Create/Replace File(file path (use dialog)="Experiment File", operation (0:open)=T8."replace or create") -> (refnum out=w550:refnum<file>)  [unwired: 4 in, 2 out]
        n201 = Write to Text File(file (use dialog)=w550, text="{\n\"frames\" : \n[\n") -> (refnum out=w548:refnum<file>)  [unwired: 2 in, 2 out]
        n202 = Bundle By Name(cluster=w553, "refnum out"=w548) -> (w552:T9)
        n203 = call <vilib>:"Add State(s) to Queue__jki_lib_state_machine.vi"("State(s) in (\"\")"=w557) -> ("States Out"=w556:string)  [unwired: 14 in]
      }
      frame "IO: Write Frame" {
        n204 = Unbundle By Name(w568) -> ("Mouse Data"=w567:T5, "refnum out"=w566:refnum<file>, "Mouse Data.Frame ID"=w559:i16)
        n205 = Not Equal?(x=w559, y=i16 1) -> (x != y?=w565:bool)
        n206 = call "Cluster to JSON.vi"("Mouse Data"=w567) -> ("JSON"=w561:string)  [unwired: 9 in, 1 out]
        n207 = Select(t=",\n", s=w565, f="") -> (s? t:f=w562:string)
        n208 = Concatenate Strings(w562, w561) -> (w560:string)
        "concatenated string 2" <- w560
        n209 = Write to Text File(file (use dialog)=w566, text=w560) -> ()  [unwired: 2 in, 3 out]
        n210 = call <vilib>:"Add State(s) to Queue__jki_lib_state_machine.vi"("State(s) in (\"\")"=w571) -> ("States Out"=w570:string)  [unwired: 14 in]
      }
      frame "IO: Close File" {
        n211 = control-ref of="Experiment Metadata"() -> (w575:refnum<vi>)
        n212 = property on="Property Node" class="MCListbox (strict)"(reference=w575) -> ("ItemNames"=w583:string[][])  [unwired: 1 in, 2 out]
        n213 = Unbundle By Name(w586) -> ("refnum out"=w584:refnum<file>)
        n214 = Write to Text File(file (use dialog)=w584, text="\n]") -> (refnum out=w573:refnum<file>)  [unwired: 2 in, 2 out]
        n215 = Index Array(array=w583, index (col)=0 ("disabled index (col)")) -> (element=w580:string[])  [unwired: 1 in]
        n216 = Index Array(array=w583, index (col)=1 ("disabled index (col)")) -> (element=w579:string[])  [unwired: 1 in]
        n217 = for {
          tunnel: w580 -> [w592] mode=indexing
          tunnel: w579 -> [w591] mode=indexing
          shift-right: [w598] -> w577
          shift-left: ",\n\"metadata\": {\n" -> [w599]
          i -> [w596]
          n218 = call "Key and Value Strings to JSON Row.vi"("Value"=w591, "Key"=w592) -> ("resulting string"=w590:string)  [unwired: 9 in]
          n219 = Not Equal To 0?(x=w596) -> (x != 0?=w597:bool)
          n220 = Select(t=", \n", s=w597, f="") -> (s? t:f=w595:string)
          n221 = Concatenate Strings(w599, w595, w590) -> (w598:string)
        }
        n222 = Concatenate Strings(w577, "\n}\n}") -> (w574:string)
        "Experiment Metadata" <- w574
        n223 = Write to Text File(file (use dialog)=w573, text=w574) -> (refnum out=w572:refnum<file>)  [unwired: 2 in, 2 out]
        n224 = Close File(refnum=w572) -> ()  [unwired: 1 in, 2 out]
        n225 = call <vilib>:"Add State(s) to Queue__jki_lib_state_machine.vi"("State(s) in (\"\")"=w589) -> ("States Out"=w588:string)  [unwired: 14 in]
      }
    }
  }
